vi "Control Experiment.vi"(8 "Error In":errorcluster, 9 "KH":T5={"KH #"=[0, 1, 2, 3, 4, 5, 6, 7, 8, 9, 10, 11, 12, 13, 14, 15], "KH Configuration"=[enum."SE+ (-gnd)", enum."SE+ (-gnd)", enum."Differential", enum."Differential", enum."SE+ (-gnd)", enum."Differential", enum."Differential", enum."SE+ (-gnd)", enum."Differential", enum."Differential", enum."SE+ (-gnd)", enum."SE+ (-gnd)", enum."Differential", enum."Ground", enum."Ground", enum."Ground"], "KH Gain"=[enum."1000x", enum."1000x", enum."1000x", enum."1000x", enum."1000x", enum."1000x", enum."1000x", enum."1000x", enum."1000x", enum."1000x", enum."1000x", enum."1000x", enum."1000x", enum."100x", enum."100x", enum."100x"], "KH Shunt Resistor"=[enum."Open", enum."Open", enum."5k Ohms", enum."5k Ohms", enum."Open", enum."5k Ohms", enum."5k Ohms", enum."Open", enum."5k Ohms", enum."5k Ohms", enum."Open", enum."Open", enum."50k Ohms", enum."Open", enum."Open", enum."Open"]} {"KH #" items=["A 1", "A 2", "A 3", "A 4", "A 5", "A 6", "A 7", "A 8", "B 1", "B 2", "B 3", "B 4", "B 5", "B 6", "B 7", "B 8"]}, 10 "Lockin":T7={"AI"=[1, 2, 3, 4, 5, 6, 7, 8, 9, 10, 11, 12, 13, 14, 15, 16], "Electrode"=["4", "5", "6", "7", "9", "11", "12", "13", "16", "17", "20", "21", "1", "", "", ""], "Label"=[8, 8, 9, 9, 8, 9, 9, 8, 2, 1, 3, 4, 6, 0, 0, 0], "Electrode Config"=[enum."Voltage (SE)", enum."Voltage (SE)", enum."Current", enum."Current", enum."Voltage (SE)", enum."Current", enum."Current", enum."Voltage (SE)", enum."Current", enum."Current", enum."Voltage (SE)", enum."Voltage (SE)", enum."Gate", enum."Ground", enum."Ground", enum."Ground"]} {"Label" items=["", "I+", "I-", "V1+", "V1-", "dV1", "Vsg", "Vbg", "V2", "I2", "I3", "V3"]}) -> (0 "Error Out":errorcluster)   [LabVIEW 2016, in "Control Experiment SM.lvclass"]
doc: "Use this VI to help configure your experiment.\n1. Choose Pickering or Not Pickering\n2. Configure the Electrode control to show which electrode is connected to which lockin\n3. Choose a Label for each electrode to configure Krohn Hite amplifier automatically\n4. Easily set all Krohn Hite channels to be \"all ground\" or \"all differential\" mode\n5. Fill out information about you and your device in the lower left corner\n6. When you are finished, or when you want to update the amplifiers, click the \"CREATE OUTPUT\" button located in upper right. Clicking this button will set the amplifiers, Pickering switch (if you have one), and write information to a functional global variable that you can easily read from elsewhere in your program"
uses:
  Control Experiment SM.lvclass
  <vilib>/addons/_JKI.lib/Serialization/JSON/JKI JSON Serialization.lvlib
  Typedefs/KH Mode-enum.ctl
  <userlib>/LevyLab/Krohn Hite 7008/typedefs/Gain-Enum.ctl
  <userlib>/LevyLab/Krohn Hite 7008/Instrument.KH7008.lvclass
  <userlib>/LevyLab/Krohn Hite 7008/typedefs/Shunt-Enum.ctl
  <userlib>/LevyLab/Krohn Hite 7008/typedefs/Input Configuration-Enum.ctl
  <vilib>/addons/_JKI.lib/REST Client/classes/REST Client/HTTP Header.ctl
  <vilib>/addons/_JKI.lib/REST Client/classes/REST Client/REST Client.lvclass
  <vilib>/JKI/JKI SMO/SMO/SMO.lvclass
  Typedefs/Control Experiment JSON--cluster.ctl
  <vilib>/Utility/sysdir.llb/System Directory Type.ctl
  <userlib>/LevyLab/Levylab Instruments/SMOs/Configuration/Configuration.lvclass
  Typedefs/Instrument--enum.ctl
  Typedefs/UI Controls --cluster.ctl
  <userlib>/_OpenG.lib/array/array.llb/Remove Duplicates from 1D Array (Variant)__ogtk.vi
  <userlib>/LevyLab/Krohn Hite 7008/typedefs/Channel-Enum.ctl
  <userlib>/LevyLab/Krohn Hite 7008/typedefs/Filter-Enum.ctl
  <userlib>/LevyLab/Krohn Hite 7008/typedefs/Coupling-Enum.ctl
  <userlib>/LevyLab/Krohn Hite 7008/typedefs/SetAll-Cluster.ctl
  <userlib>/LevyLab/Krohn Hite 7008/typedefs/SetAll-Array.ctl
  <userlib>/LevyLab/Levylab Instruments/SMOs/Logger.PGSQL/Logger.PGSQL.lvclass
  <userlib>/LevyLab/Lockin-Multichannel/Instrument.Lockin/Instrument.Lockin.lvclass
  <userlib>/LevyLab/Levylab Instruments/Instrument Types/CBridge/Instrument.CBridge.lvclass
  <userlib>/LevyLab/Levylab Instruments/Instrument Types/Strain/Instrument.Strain.lvclass
  <userlib>/_MGI/File/MGI Create Directory Chain Behavior Enum.ctl
  C:/Program Files (x86)/National Instruments/LabVIEW 2016/user.lib/LevyLab/Levylab Instruments/SMOs/Logger/Logger.lvclass
  C:/Program Files (x86)/National Instruments/LabVIEW 2016/vi.lib/JKI/JKI SMO/SMO/SMO.lvclass
panel:
  in  "I'm Finished Taking Data!":bool
  out "Values have changed":bool=TRUE
  in  "Create Output":bool
  in  "OK":bool
  out "Control Experiment":refnum<class "Control Experiment SM.lvclass">
  in  "C.E.":refnum<class "Control Experiment SM.lvclass">
  in  "Tab Control":T1(tab)=enum."Sandbox"
  in  "DC Coupled":bool=TRUE
  in  "Bandwidth Filter":bool=TRUE
  in  "#AO":u32=8
  in  "Gain":dbl[](array[numeric])=[1.0, 1.0, 1.0, 1.0, 1.0, 1.0, 1.0, 1.0, 1.0, 1.0, 1.0, 1.0, 1.0, 1.0, 1.0, 1.0]
  in  "#AI":u32=16
  in  "KH All Buttons":T8(radio)
  in  "Defualt Shunt Resistor":T4=enum."5k Ohms"
  in  "Description":string="    devices:\n    \n    1. 80x80um rectangle\n    2. hash: 200 horizontal and vertical lines 400nm apart\n    3. hash structures: 400, 200nm apart horizontal and vertical lines"
  in  "Sample (SAXXXX)":string="SA40178"
  in  "Device (YYYYMMDD)":string="20210125"
  in  "Instrument":T9=enum."MNK"
  in  "Username":string="Aditi"
  in  "non KH":T10 {"Labels 2" items=["", "I+", "I-", "V1+", "V1-", "dV1", "Vsg", "Vbg", "V2", "I2", "I3", "V3"]}
  in  "Strain Cell Address":refnum<visa-resource-name>
  in  "Capacitance Bridge Address":refnum<visa-resource-name>
  in  "C Bridge?":bool
  in  "Strain Cell?":bool
  in  "Krohn Hite?":bool=TRUE
  in  "KH Addresses":refnum<visa-resource-name>[](array[refnum])=["COM20", "COM14"] caption="KH Address[A,B,C,...]"
  in  "Lockin Address":string
  in  "Ring":u16(ring)=2 items=["----Sweep Control----", "Sweep Control.vi", "Continuous B Sweep.vi", "----Transport----", "IV.vi", "IV_Sweep.vi", "Lockin_time.vi", "Lockin_Vsg.vi", "Lockin_sweep.vi", "Lockin_AIWFM_time.vi", "THz_TimeDelay.vi", "Sweep_AIWFM_time.vi"]
  in  "Open VI":bool
  in  "Open Lockin":bool
  in  "Write Pickering Config":bool
  in  "Read Pickering Config":bool
  out "Refresh Token Out":string="0/0ccae0b202a2d5ce21e5be9cd72246b8"
  in  "Default Path":path=path "D:/Data" caption="Default Path (Do not add your instrument name here)(Typ. G:\\My Drive\\ansom\\Data)"
  out "Comments":string="Device: \r  Device Name: SA40178.20210125\r  Computer: KHOLEK\r  User: Aditi\r  Instrument: MNK\r  Description: |\r        devices:\r        \r        1. 80x80um rectangle\r        2. hash: 200 horizontal and vertical lines 400nm apart\r        3. hash structures: 400, 200nm apart horizontal and vertical lines\r\rExperiment: \r  Time: 2021-02-22T11:02:02\r  Description: |\r\rSweep: \r- Loop1: [OFF, 0.000000]\r- Loop2: [OFF, 0.000000]\r- Loop3: [OFF, 0.000000]\r- Loop4: [OFF, 0.000000]\r\rWiring: \r- Electrode 4: Lockin 1, V2, KH1 Channel 1, SE+ (-gnd), 1000x, Open\r- Electrode 5: Lockin 2, V2, KH1 Channel 2, SE+ (-gnd), 1000x, Open\r- Electrode 6: Lockin 3, I2, KH1 Channel 3, Differential, 1000x, 5k Ohms\r- Electrode 7: Lockin 4, I2, KH1 Channel 4, Differential, 1000x, 5k Ohms\r- Electrode 9: Lockin 5, V2, KH1 Channel 5, SE+ (-gnd), 1000x, Open\r- Electrode 11: Lockin 6, I2, KH1 Channel 6, Differential, 1000x, 5k Ohms\r- Electrode 12: Lockin 7, I2, KH1 Channel 7, Differential, 1000x, 5k Ohms\r- Electrode 13: Lockin 8, V2, KH1 Channel 8, SE+ (-gnd), 1000x, Open\r- Electrode 16: Lockin 9, I-, KH2 Channel 1, Differential, 1000x, 5k Ohms\r- Electrode 17: Lockin 10, I+, KH2 Channel 2, Differential, 1000x, 5k Ohms\r- Electrode 20: Lockin 11, V1+, KH2 Channel 3, SE+ (-gnd), 1000x, Open\r- Electrode 21: Lockin 12, V1-, KH2 Channel 4, SE+ (-gnd), 1000x, Open\r- Electrode 1: Lockin 13, Vsg, KH2 Channel 5, Differential, 1000x, 50k Ohms\r\rLockin: \r  AO: \r  - AO 1: amp = 0.000 mV, DC = 0.000 mV, f = 1.00 Hz, phi = 0.00°, Triangle\r  - AO 2: amp = 0.000 mV, DC = 0.000 mV, f = 1.00 Hz, phi = 0.00°, Triangle\r  - AO 3: amp = 0.000 mV, DC = 0.000 mV, f = 1.00 Hz, phi = 0.00°, Triangle\r  - AO 4: amp = 0.000 mV, DC = 0.000 mV, f = 1.00 Hz, phi = 0.00°, Triangle\r  - AO 5: amp = 0.000 mV, DC = 0.000 mV, f = 1.00 Hz, phi = 0.00°, Triangle\r  - AO 6: amp = 10.000 mV, DC = 0.000 mV, f = 1.00 Hz, phi = 0.00°, Triangle\r  - AO 7: amp = 0.000 mV, DC = 0.000 mV, f = 1.00 Hz, phi = 0.00°, Triangle\r  - AO 8: amp = 0.000 mV, DC = 0.000 mV, f = 1.00 Hz, phi = 0.00°, Triangle\r  - AO 9: amp = 0.000 mV, DC = 0.000 mV, f = 1.00 Hz, phi = 0.00°, Triangle\r  - AO 10: amp = 10.000 mV, DC = 0.000 mV, f = 1.00 Hz, phi = 0.00°, Triangle\r  - AO 11: amp = 0.000 mV, DC = 0.000 mV, f = 1.00 Hz, phi = 0.00°, Triangle\r  - AO 12: amp = 0.000 mV, DC = 0.000 mV, f = 1.00 Hz, phi = 0.00°, Triangle\r  - AO 13: amp = 0.000 mV, DC = 0.000 mV, f = 1.00 Hz, phi = 0.00°, Sine\r  - AO 14: amp = 0.000 mV, DC = 0.000 mV, f = 1.00 Hz, phi = 0.00°, Sine\r  - AO 15: amp = 0.000 mV, DC = 0.000 mV, f = 1.00 Hz, phi = 0.00°, Sine\r  - AO 16: amp = 0.000 mV, DC = 0.000 mV, f = 1.00 Hz, phi = 0.00°, Sine\r  - AO 17: amp = 0.000 mV, DC = -0.000 mV, f = 1.00 Hz, phi = 0.00°, Sine\r  - AO 18: amp = 0.000 mV, DC = 0.000 mV, f = 1.00 Hz, phi = 0.00°, Sine\r  - AO 19: amp = 0.000 mV, DC = 0.000 mV, f = 1.00 Hz, phi = 0.00°, Sine\r  - AO 20: amp = 0.000 mV, DC = 0.000 mV, f = 1.00 Hz, phi = 0.00°, Sine\r  - AO 21: amp = 0.000 mV, DC = 0.000 mV, f = 1.00 Hz, phi = 0.00°, Sine\r  - AO 22: amp = 0.000 mV, DC = 0.000 mV, f = 1.00 Hz, phi = 0.00°, Sine\r  - AO 23: amp = 0.000 mV, DC = 0.000 mV, f = 1.00 Hz, phi = 0.00°, Sine\r  - AO 24: amp = 0.000 mV, DC = 0.000 mV, f = 1.00 Hz, phi = 0.00°, Sine\r  REF: \r  - Lockin 1: f = 1.00 Hz, phi = 0.00°, TC = 0.10 s, order = 2 \r  Sampling: \r  - Fs: 10000.000000\r  - N: 1000\r"
  out "Device Folder":path=path "D:/Data/MNK/SA40178.20210125" caption="(\\base path\\project\\device\\ )"
  out "JSON String":string="{\r\n    \"Device\":{\r\n        \"Device\":\"SA40178.20210125\",\r\n        \"User\":\"Aditi\",\r\n        \"Time\":\"2021-02-22T11:02:02\",\r\n        \"Computer Name\":\"KHOLEK\"\r\n    },\r\n    \"Wiring\":{\r\n        \"Lockin Ch\":[\r\n            1,\r\n            2,\r\n            3,\r\n            4,\r\n            5,\r\n            6,\r\n            7,\r\n            8,\r\n            9,\r\n            10,\r\n            11,\r\n            12,\r\n            13,\r\n            14,\r\n            15,\r\n            16\r\n        ],\r\n        \"KH Electrodes\":[\r\n            \"4\",\r\n            \"5\",\r\n            \"6\",\r\n            \"7\",\r\n            \"9\",\r\n            \"11\",\r\n            \"12\",\r\n            \"13\",\r\n            \"16\",\r\n            \"17\",\r\n            \"20\",\r\n            \"21\",\r\n            \"1\",\r\n            \"\",\r\n            \"\",\r\n            \"\"\r\n        ],\r\n        \"KH Labels\":[\r\n            \"V2\",\r\n            \"V2\",\r\n            \"I2\",\r\n            \"I2\",\r\n            \"V2\",\r\n            \"I2\",\r\n            \"I2\",\r\n            \"V2\",\r\n            \"I-\",\r\n            \"I+\",\r\n            \"V1+\",\r\n            \"V1-\",\r\n            \"Vsg\",\r\n            \"\",\r\n            \"\",\r\n            \"\"\r\n        ],\r\n        \"Other Electrodes\":[\r\n            \"4\",\r\n            \"5\",\r\n            \"6\",\r\n            \"7\",\r\n            \"9\",\r\n            \"11\",\r\n            \"12\",\r\n            \"13\",\r\n            \"16\",\r\n            \"17\",\r\n            \"20\",\r\n            \"21\",\r\n            \"1\",\r\n            \"\",\r\n            \"\",\r\n            \"\"\r\n        ],\r\n        \"Other Labels\":[\r\n            \"V2\",\r\n            \"V2\",\r\n            \"I2\",\r\n            \"I2\",\r\n            \"V2\",\r\n            \"I2\",\r\n            \"I2\",\r\n            \"V2\",\r\n            \"I-\",\r\n            \"I+\",\r\n            \"V1+\",\r\n            \"V1-\",\r\n            \"Vsg\",\r\n            \"\",\r\n            \"\",\r\n            \"\"\r\n        ]\r\n    }\r\n}"
  in  "Labels Strings":string[](array[string])=["", "I+", "I-", "V1+", "V1-", "dV1", "Vsg", "Vbg", "V2", "I2", "I3", "V3"]
  out "YAML example":string="description: This is a dummy dataset which mimics smFRET data.\n\nsetup:\n    ## Mandatory fields\n    num_pixels: 2                # using 2 detectors\n    num_spots: 1                 # a single confocal excitation\n    num_spectral_ch: 2           # donor and acceptor detection\n    num_polarization_ch: 1       # no polarization selection\n    num_split_ch: 1              # no beam splitter\n    modulated_excitation: False  # CW excitation, no modulation\n    lifetime: False              # no TCSPC in detection\n\n    ## Optional fields\n    excitation_wavelengths:      # List of excitation wavelenghts\n       - !!float 532e-9\n    excitation_cw:               # List of booleans, True if wavelength is CW\n       - True\n    detection_wavelengths:       # Nominal center wavelength for each for detection ch\n       - !!float 580e-9\n       - !!float 640e-9\n\nsample:\n  sample_name: describe the sample here\n  buffer_name: describe the buffer here\n  dye_names: 'Cy3B, ATTO647N'   # Comma separates names of fluorophores\n\nidentity:\n    author: Author Name\n    author_affiliation: Name of Research Institution\n\nprovenance:\n    filename: 'photon_data.hdf5'\n    software: Acquisition Software Name\n\nphoton_data:\n    timestamps_specs:\n        timestamps_unit: !!float 10e-9  # 10 ns\n    measurement_specs:\n        measurement_type: smFRET\n        detectors_specs:\n            spectral_ch1: [0]  # list of donor's detector IDs\n            spectral_ch2: [1]  # list of acceptor's detector IDs"
  in  "String":string
  # "SANDBOX:"
  # "Sample"
  # "Krohn Hite"
  # "Lockin"
  # "Lockin"
  # "Krohn Hite"
  # "Other"
  # "Device and Project Description"
  # "Hardware Configuration"
  # "Experiment VIs"
  # "Lockin (Local)"
  # "Path Configuration"
  # "Use this VI to help configure your experiment.\n1. Choose Pickering or Not Pickering\n2. Configure the Electrode control to show which electrode is connected to which lockin\n3. Choose a Label for each electrode to configure Krohn Hite amplifier automatically\n4. Easily set all Krohn Hite channels to be \"all ground\" or \"all differential\" mode\n5. Fill out information about you and your device in the lower left corner\n6. When you are finished, or when you want to update the amplifiers, click the \"CREATE OUTPUT\" button located in upper right.\nClicking this button will set the amplifiers, Pickering switch (if you have one), and write information to a functional global variable that you can easily read from elsewhere in your program"
  # "If you want to have new labels for the \"Labels\" field you can type them here"
  # "The magic words are:\nI\nVsg\nVbg\ndV\nV"
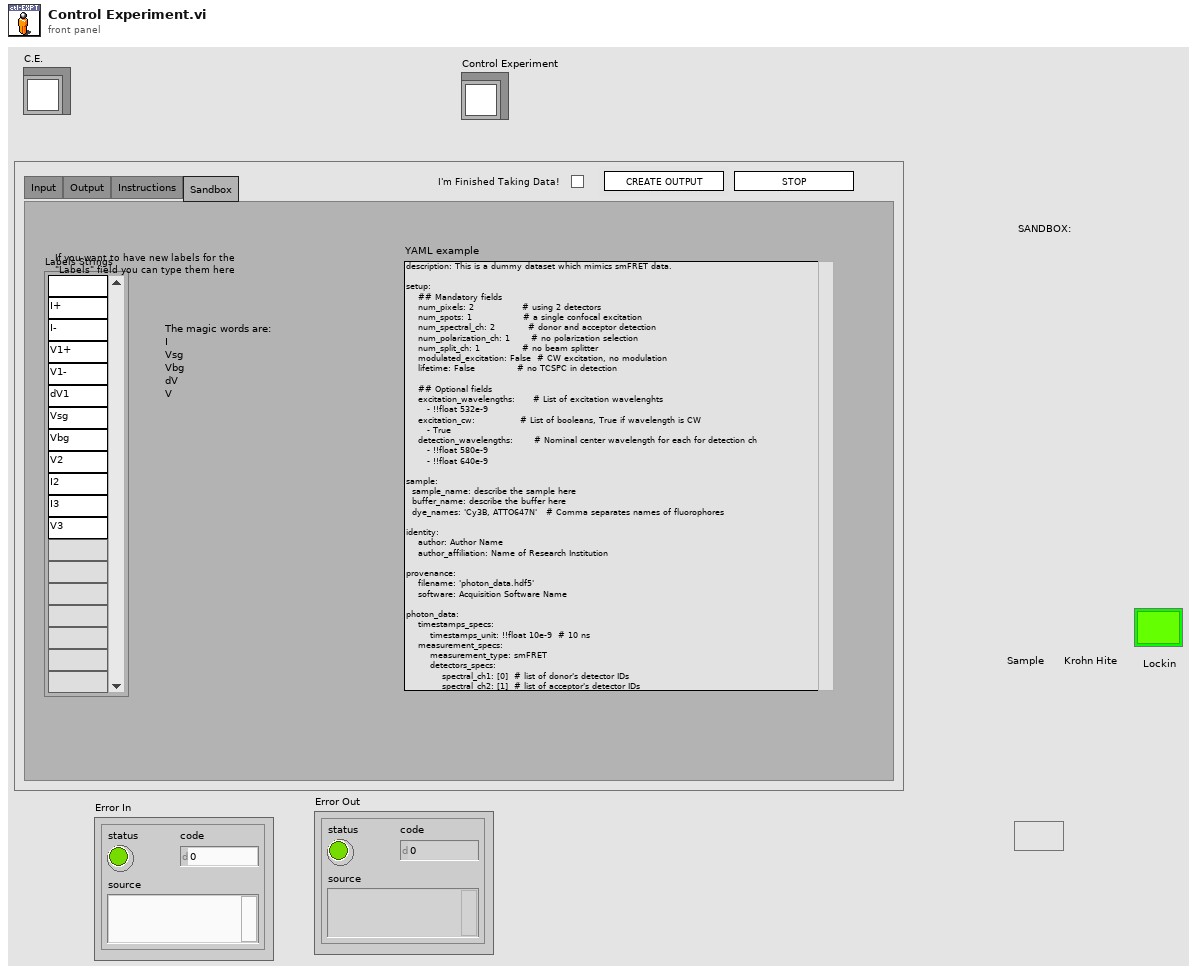
[diagram p1: front panel]
types:
  T1 = enum32{"Input", "Pickering", "Output", "Instructions", "Sandbox"}
  T2 = typedef "Instrument.KH7008.lvclass/Input Configuration-Enum.ctl" = enum16{"Ground", "SE+ (-gnd)", "SE- (+gnd)", "Differential"}
  T3 = typedef "Instrument.KH7008.lvclass/Gain-Enum.ctl" = enum16{"1x", "10x", "100x", "1000x"}
  T4 = typedef "Instrument.KH7008.lvclass/Shunt-Enum.ctl" = enum16{"Open", "50 Ohms", "500 Ohms", "5k Ohms", "50k Ohms", "10M Ohm"}
  T5 = cluster{"KH #":u16[], "KH Configuration":T2[], "KH Gain":T3[], "KH Shunt Resistor":T4[]}
  T6 = typedef "Control Experiment SM.lvclass/KH Mode-enum.ctl" = enum16{"Ground", "Current", "Voltage (SE)", "Voltage (Diff)", "Gate"}
  T7 = cluster{"AI":u32[], "Electrode":string[], "Label":u16[], "Electrode Config":T6[]}
  T8 = enum32{"No Selection", "All Ground", "All Differential"}
  T9 = typedef "Control Experiment SM.lvclass/Instrument--enum.ctl" = enum16{"----- AFM/EBL -----", "AGILENT", "CYPHER", "Gemini2", "JEOL", "MFP3D", "----- Cryostat -----", "CF900", "DR200", "MNK", "PPMS 1", "PPMS 2", "PPMS 3", "----- Optics -----", "THz 1", "THz 2"}
  T10 = cluster{"Scroll Bar":string[], "Electrodes 2":string[], "Labels 2":u16[], "unused":string[]}
  T11 = enum16{"A 1", "A 2", "A 3", "A 4", "A 5", "A 6", "A 7", "A 8", "B 1", "B 2", "B 3", "B 4", "B 5", "B 6", "B 7", "B 8", "none"}
  T12 = enum32{"invalid app kind", "Development System", "Run Time System", "Student Edition", "Embedded LabVIEW", "Evaluation", "Custom"}
  T13 = enum32{"Bad", "Idle", "Run top level", "Running"}
  T14 = enum32{"Invalid", "Standard", "Closed", "Hidden", "Minimized", "Maximized"}
  T15 = typedef "MGI Create Directory Chain Behavior Enum.ctl" = enum16{"Auto Detect", "Path Contains a File", "Path Does Not Contain a File"}
  T16 = typedef "Instrument.KH7008.lvclass/SetAll-Cluster.ctl" = cluster{"Channel":T17, "Gain":T3, "Bandwidth Filter":T18, "Shunt Resistor":T4, "Coupling":T19, "Input Config":T2}
  T17 = typedef "Instrument.KH7008.lvclass/Channel-Enum.ctl" = enum16{"Channel 1", "Channel 2", "Channel 3", "Channel 4", "Channel 5", "Channel 6", "Channel 7", "Channel 8"}
  T18 = typedef "Instrument.KH7008.lvclass/Filter-Enum.ctl" = enum16{"OFF", "ON"}
  T19 = typedef "Instrument.KH7008.lvclass/Coupling-Enum.ctl" = enum16{"AC", "DC"}
  T20 = enum16{"GSR", "Research Projects", "Undergrads", "Researchers", "Hardware", "Software", "LevyLab", "Samples", "Manuscripts", "AoT", "WorkStudy"}
  T21 = enum16{"A 1", "A 2", "A 3", "A 4", "A 5", "A 6", "A 7", "A 8", "B 1", "B 2", "B 3", "B 4", "B 5", "B 6", "B 7", "B 8", "none"}[]
  T22 = typedef "Control Experiment SM.lvclass/Experiment Description--cluster.ctl" = cluster{"User":string, "Device":string, "Device Path":path, "Device Description":string, "Experiment Path":path, "Experiment Description":string, "Instrument":T9, "Device Description (JSON)":string, "Experiment Description (JSON)":string, "Comments":string, "Sweep":cluster{"key":string, "value":variant}[]}
  T23 = typedef "Control Experiment SM.lvclass/Wiring Description--cluster.ctl" = cluster{"AI":cluster{"Channel":u32, "Gain":dbl}, "Device":cluster{"Electrode":string, "Label":string, "Type":string}, "KH":cluster{"Channel":string, "Configuration":string, "Gain":u32, "Shunt Resistor":u32}, "AO":cluster{"Channel":u32, "Gain":dbl}}[]
  T24 = typedef "Instrument.KH7008.lvclass/SetAll-Array.ctl" = T16[]
  T25 = typedef "Control Experiment SM.lvclass/UI Controls --cluster.ctl" = cluster{"Sample":string, "Device":string, "Username":string, "Description":string, "Default Path":path, "AWS Path":path, "Instrument":T9, "Lockin?":bool, "Lockin Address":string, "Krohn Hite?":bool, "KH Addresses":refnum<visa-resource-name>[], "KH All Buttons":enum32{"No Selection", "All Ground", "All Differential"}, "Strain Cell?":bool, "Strain Cell Address":refnum<visa-resource-name>, "C Bridge?":bool, "Capacitance Bridge Address":refnum<visa-resource-name>, "Lockin":cluster{"AI":u32[], "Electrode":string[], "Label":u16[], "Electrode Config":T6[]}, "KH":cluster{"KH #":enum16{"A 1", "A 2", "A 3", "A 4", "A 5", "A 6", "A 7", "A 8", "B 1", "B 2", "B 3", "B 4", "B 5", "B 6", "B 7", "B 8", "none"}[], "KH Configuration":T2[], "KH Gain":T3[], "KH Shunt Resistor":T4[], "Filter":bool, "DC Coupled":bool}, "non KH":cluster{"Scroll Bar":string[], "Electrodes 2":string[], "Labels 2":u16[], "unused":string[]}, "#AI":u32}
  T26 = typedef "REST Client.lvlib/REST Client.lvclass/HTTP Header.ctl" = cluster{"header":string, "value":string}
  T27 = cluster{"Core":cluster{"Current VI Reference":refnum<vi>, "Close Panel on Exit?":bool}, "C.E.":refnum<class "Control Experiment SM.lvclass">, "Experiment":T22, "Wiring":T23, "Channel Settings":cluster{"Channel Setting":T24}[], "KH All Buttons":enum32{"No Selection", "All Ground", "All Differential"}, "Lockin":cluster{"AI":u32[], "Electrode":string[], "Label":u16[], "Electrode Config":T6[]}, "KH":cluster{"KH #":u16[], "KH Configuration":T2[], "KH Gain":T3[], "KH Shunt Resistor":T4[]}, "non KH":cluster{"Scroll Bar":string[], "Electrodes 2":string[], "Labels 2":u16[], "unused":string[]}, "UI":T25, "Asana":cluster{"Authentication Info":cluster{"Client ID":string, "Client Secret":string, "Redirect URI":string, "Token Endpoint":string, "Scope":string}, "Authentication Header":T26[], "Refresh Token":string, "Time Stamp":timestamp}, "Logger":refnum<class "Logger.PGSQL.lvclass">, "Config":refnum<class "Configuration.lvclass">, "VI paths":path[], "top level?":bool}
  T28 = cluster{"Authentication Info":cluster{"Client ID":string, "Client Secret":string, "Redirect URI":string, "Token Endpoint":string, "Scope":string}, "Authentication Header":T26[], "Refresh Token":string, "Time Stamp":timestamp}
  T29 = cluster{"Current VI Reference":refnum<vi>, "Close Panel on Exit?":bool}
  T30 = typedef "System Directory Type.ctl" = i32
  T31 = typedef "Control Experiment SM.lvclass/Control Experiment JSON--cluster.ctl" = cluster{"Device":cluster{"Device":string, "User":string, "Time":string, "Computer Name":string}, "Wiring":cluster{"Lockin Ch":u32[], "KH Electrodes":string[], "KH Labels":string[], "Other Electrodes":string[], "Other Labels":string[]}}
  T32 = cluster{"Client ID":string, "Client Secret":string, "Redirect URI":string, "Token Endpoint":string, "Scope":string}
  T33 = cluster{"gid":string, "name":string, "resource_type":string}[]
  T34 = cluster{"id":i64, "gid":string, "resource_type":string, "name":string}[]
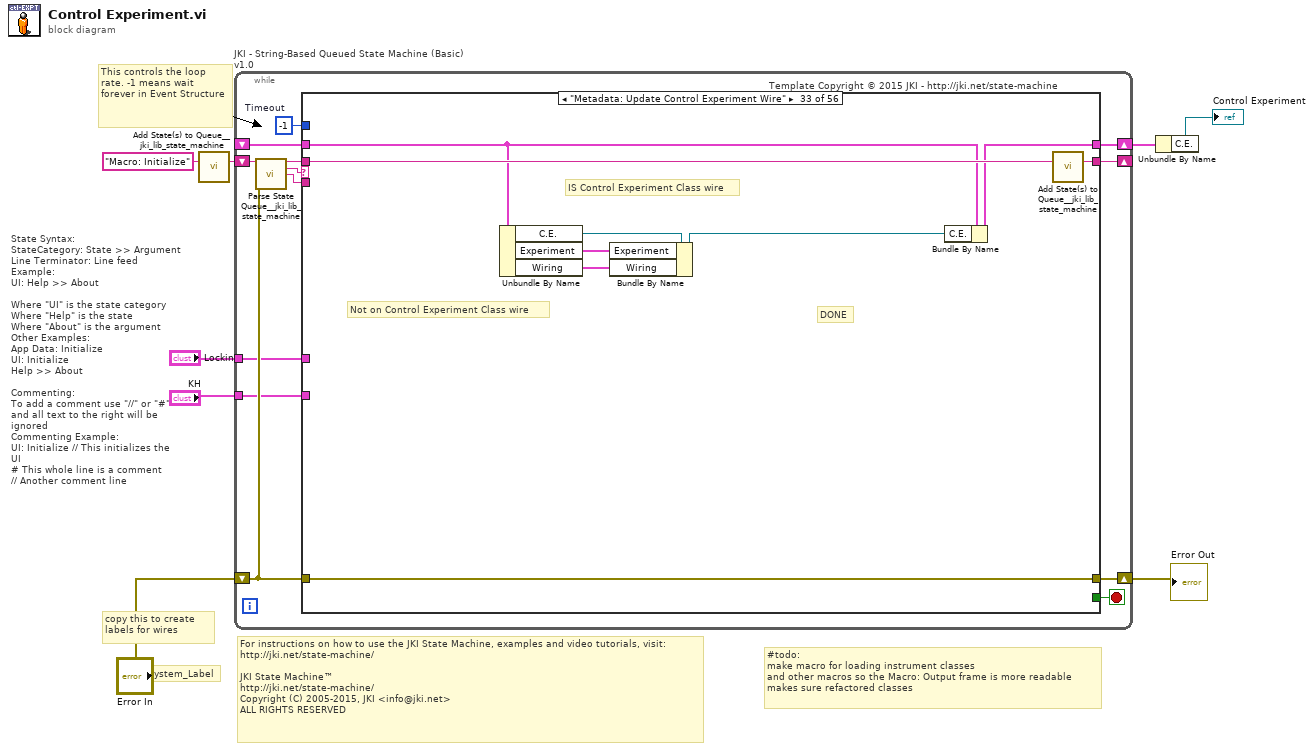
[diagram p0: block diagram]
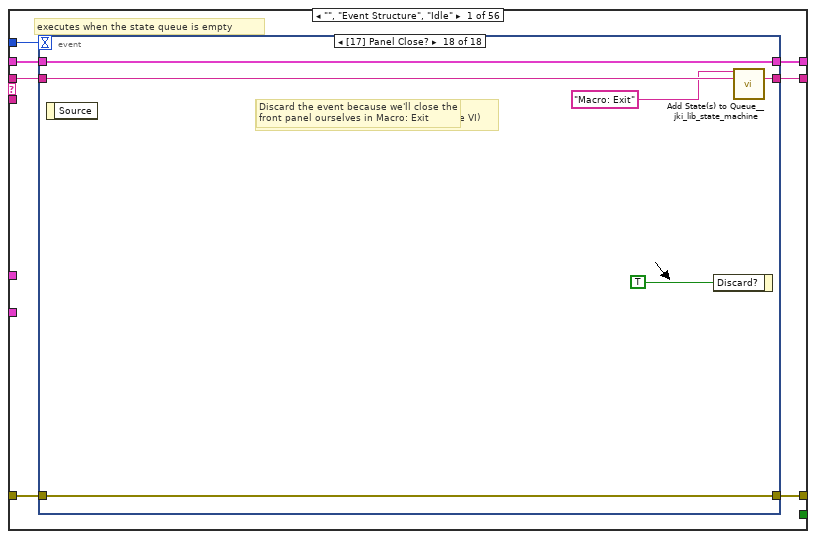
[diagram p2: hidden frame]
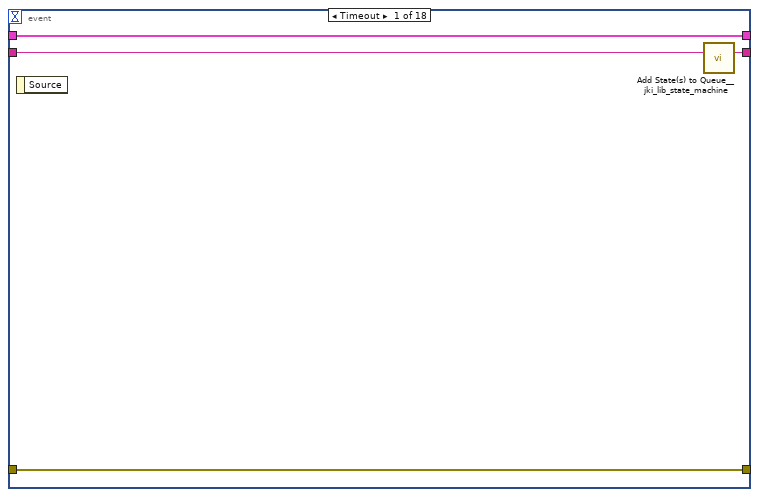
[diagram p3: hidden frame]
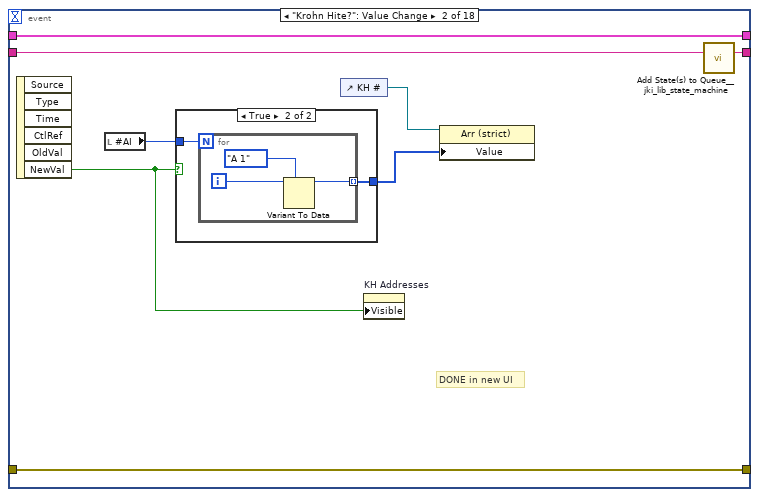
[diagram p4: hidden frame]
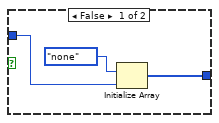
[diagram p5: hidden frame]
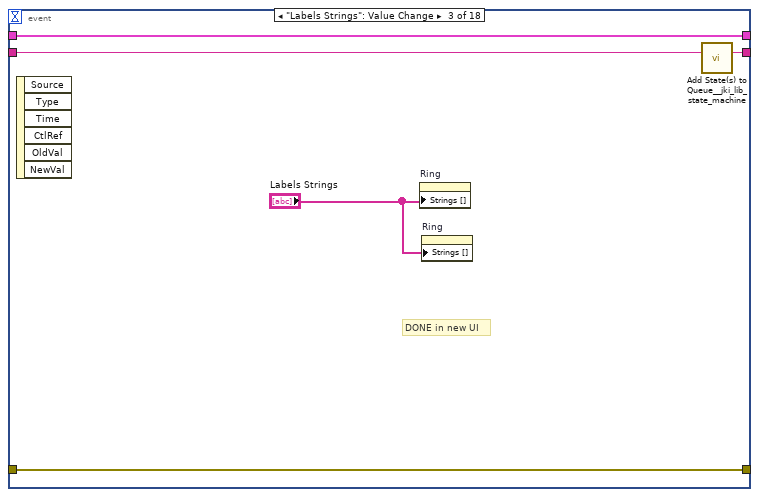
[diagram p6: hidden frame]
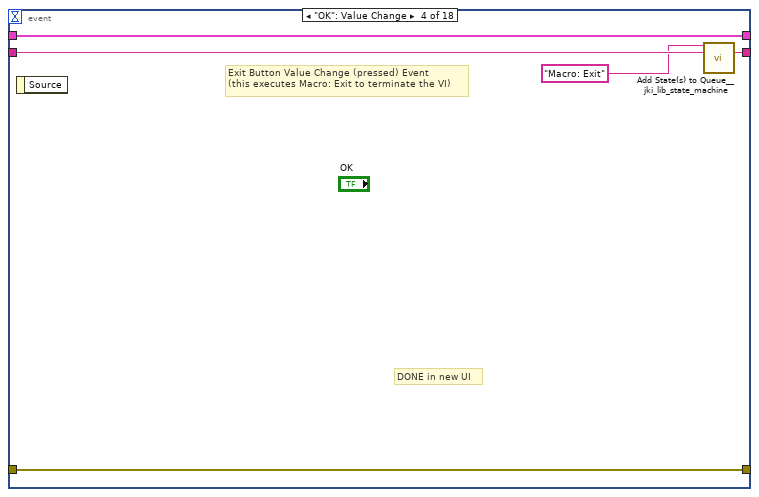
[diagram p7: hidden frame]
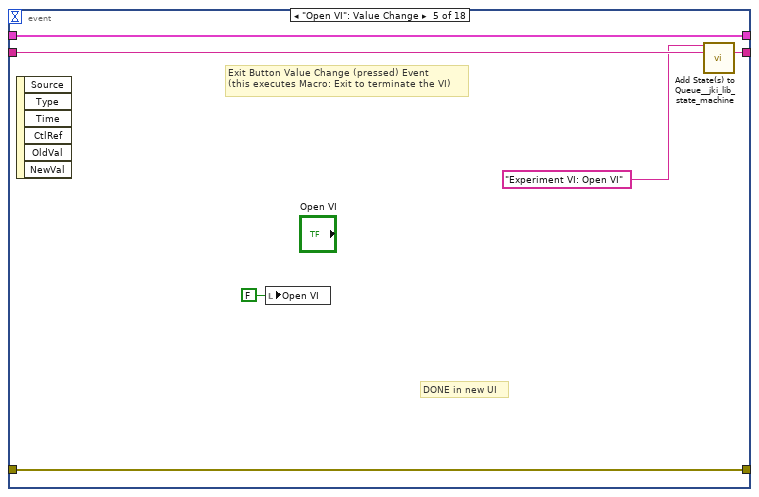
[diagram p8: hidden frame]
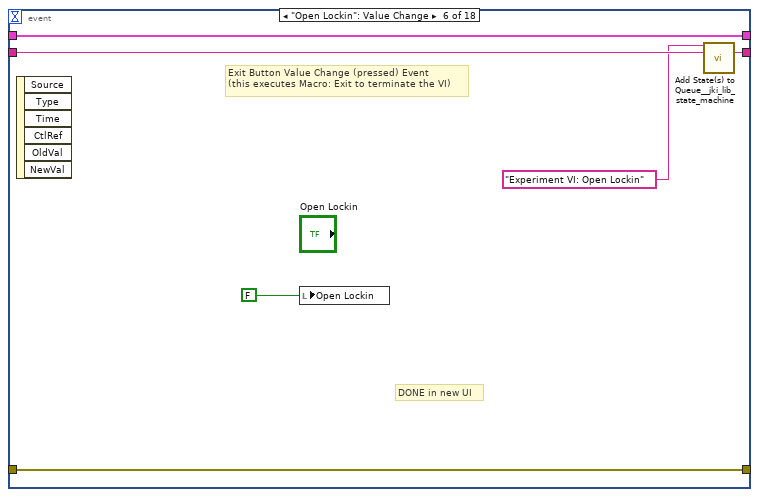
[diagram p9: hidden frame]
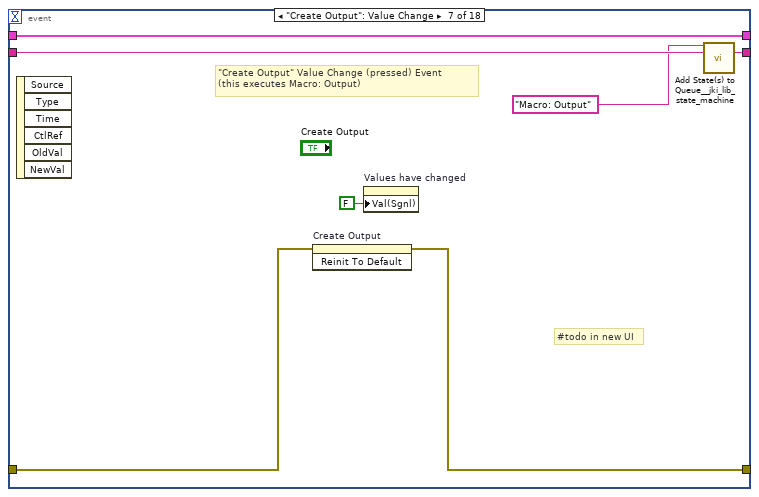
[diagram p10: hidden frame]
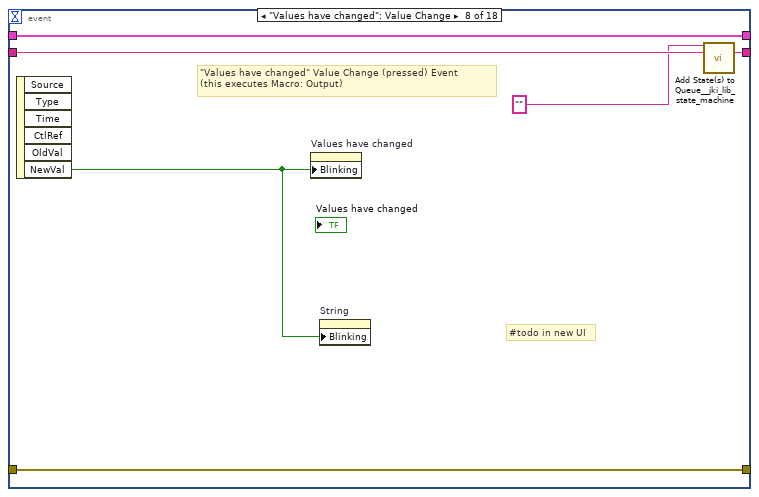
[diagram p11: hidden frame]
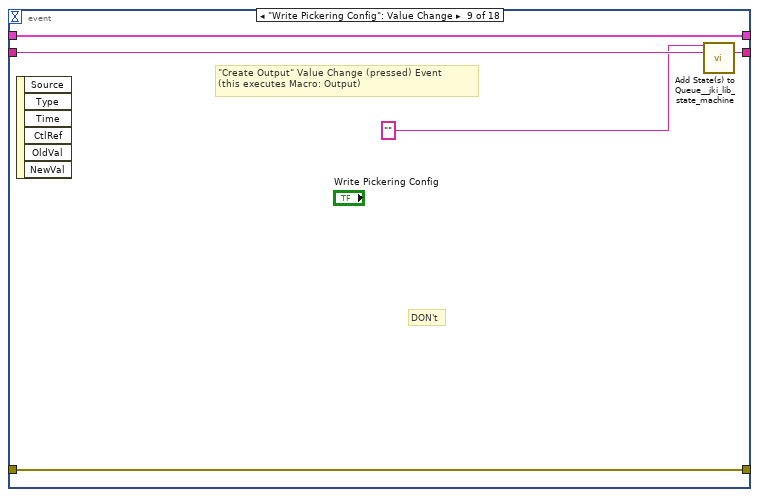
[diagram p12: hidden frame]
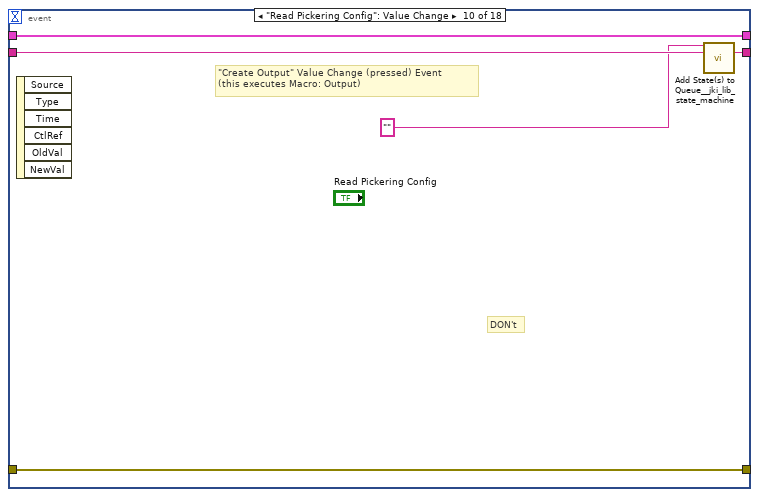
[diagram p13: hidden frame]
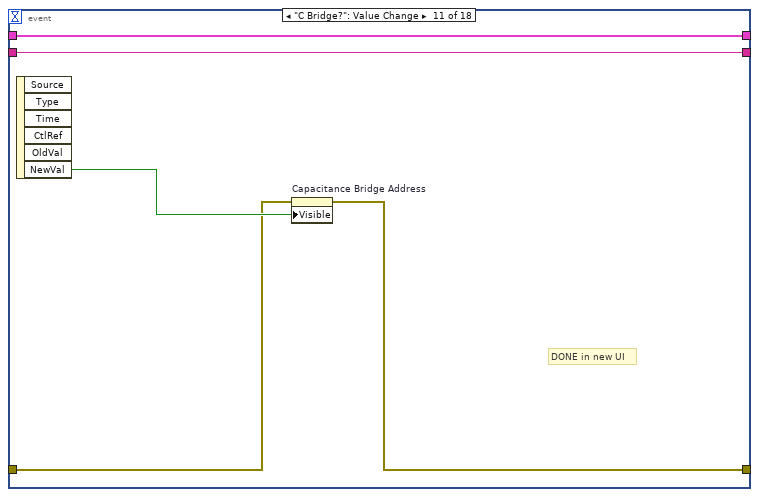
[diagram p14: hidden frame]
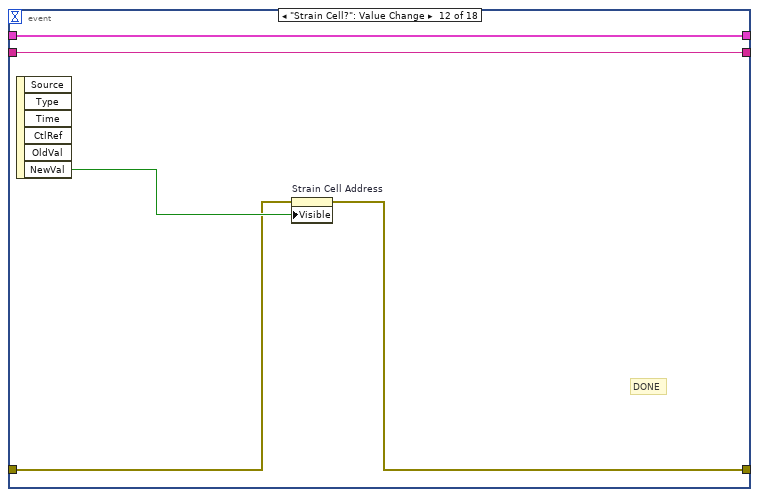
[diagram p15: hidden frame]
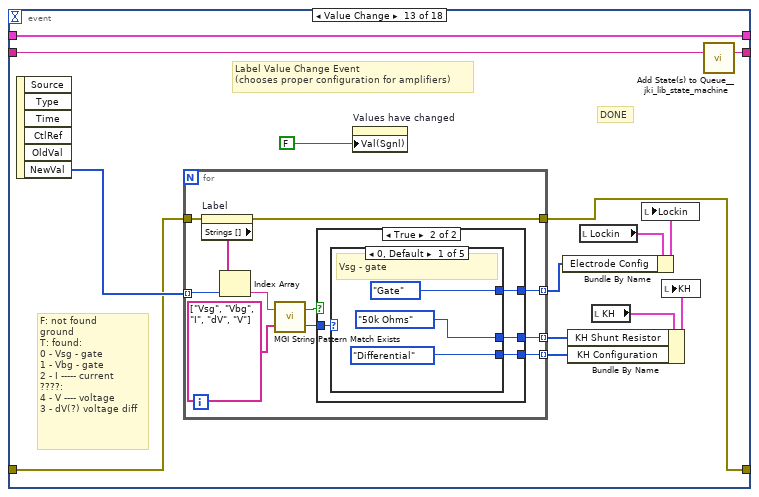
[diagram p16: hidden frame]
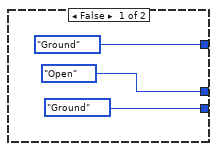
[diagram p17: hidden frame]
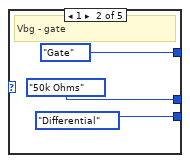
[diagram p18: hidden frame]
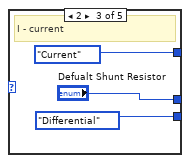
[diagram p19: hidden frame]
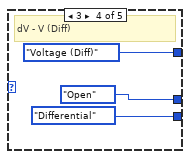
[diagram p20: hidden frame]
diagram:
  # "#todo:\nmake macro for loading instrument classes\nand other macros so the Macro: Output frame is more readable\nmakes sure refactored classes"
  # "For instructions on how to use the JKI State Machine, examples and video tutorials, visit:\nhttp://jki.net/state-machine/\n\nJKI State Machine™\nhttp://jki.net/state-machine/\nCopyright (C) 2005-2015, JKI <info@jki.net>\nALL RIGHTS RESERVED"
  # "State Syntax:\nStateCategory: State >> Argument\nLine Terminator: Line feed\nExample:\nUI: Help >> About\n\nWhere \"UI\" is the state category\nWhere \"Help\" is the state\nWhere \"About\" is the argument\nOther Examples:\nApp Data: Initialize\nUI: Initialize\nHelp >> About\n\nCommenting:\nTo add a comment use \"//\" or \"#\" and all text to the right will be ignored\nCommenting Example:\nUI: Initialize // This initializes the UI\n# This whole line is a comment\n// Another comment line"
  # "copy this to create labels for wires"
  # "This controls the loop rate. -1 means wait forever in Event Structure"
  # "System_Label"
  n1 = call <vilib>:"Add State(s) to Queue__jki_lib_state_machine.vi"("State(s) in (\"\")"="Macro: Initialize") -> ("States Out"=w8:string)  [unwired: 14 in]
  n2 = while "JKI - String-Based Queued State Machine (Basic) v1.0" {
    shift-right: [w14] -> w6
    shift-left: _ -> [w13]
    shift-right: [w17] -> w2
    shift-left: "Error In" -> [w11]
    shift-right: [w16] -> _
    shift-left: w8 -> [w18]
    tunnel: "Lockin" -> [w10]
    tunnel: "KH" -> [w9]
    stop <- w15 stop-if-true
    w12 = -1  # Timeout
    # "Template Copyright © 2015 JKI - http://jki.net/state-machine"
    n3 = call <vilib>:"Parse State Queue__jki_lib_state_machine.vi"("State Queue"=w18, "Error In (no error)"=w11) -> ("Remaining States"=w20:string, "Current State"=w21:string, "Arguments"=w19:string)  [unwired: 11 in]
    n4 = case shown="\"Metadata: Update Control Experiment Wire\"" w21 {
      selector: w21 -> [_ _ w195 _ _ _ _ _ _ _ _ _ _ _ _ _ _ _ _ _ _ _ _ _ _ _ _ _ _ _ _ _ _ _ _ _ _ _ _ _ _ _ _ _ _ _ _ _ _ _ _ _ _ _ _ _]
      tunnel: w20 -> [w28 w194 w199 w217 w223 w228 w232 w253 w264 w279 w315 w323 w327 w346 w378 w387 w398 w424 w439 w452 w456 w461 w472 w479 w492 w497 w502 w506 w518 w534 w560 w574 w583 w596 w603 w629 w633 w651 w684 w771 w786 w794 w805 w822 w837 w841 w849 w867 w898 w914 w935 w949 w954 w958 w968 w986]
      tunnel: w19 -> [_ _ _ _ _ _ _ _ _ _ _ _ _ _ _ w382 w392 _ _ _ _ _ _ _ _ _ _ _ _ _ _ _ _ _ _ _ _ _ _ _ _ _ _ _ _ _ _ _ _ _ _ _ _ _ _ _]
      tunnel: w13 -> [w26 w191 w197 w208 w220 w226 w229 _ w259 w275 w294 w318 w324 w335 w353 w385 w394 w421 w436 w450 w453 w458 w469 w477 w489 w494 w499 w503 w514 w530 w557 w572 w579 w594 w601 w620 w630 w649 w676 w764 w783 w792 w798 w818 w827 w838 w843 w851 w883 w911 w922 w947 w952 w955 w960 w984]
      tunnel: [w25 w192 w201 w214 errorcluster {"status"=FALSE, "code"=0, "source"=""} ("error out") w225 w230 w250 w262 w270 w295 w321 w325 w336 w376 w383 w395 w422 w437 w440 w454 w459 w470 w475 w490 w495 w500 w504 w516 w532 w544 w564 w576 w584 w599 w615 w631 w635 w675 w768 w784 w788 w802 w816 w828 w839 w847 w860 w880 w912 w933 w942 w950 w956 w961 w972] -> w17
      tunnel: w11 -> [w24 w192 w200 w214 w219 w225 w230 w250 w262 w276 w296 w319 w325 w344 w376 w384 w396 w422 w437 w447 w454 w459 w470 w475 w490 w495 w500 w504 w516 w532 w542 w565 w576 w585 w597 w617 w631 w645 w675 w760 w784 w787 w803 w819 w829 w839 w847 w850 w896 w912 w933 w943 w951 w956 w962 w974]
      tunnel: [w27 w193 w198 w216 w222 w227 w231 w252 w263 w278 w314 w322 w326 w345 w377 w386 w397 w423 w438 w451 w455 w460 w471 w478 w491 w496 w501 w505 w517 w533 w559 w573 w582 w595 w602 w628 w632 w650 w683 w770 w785 w793 w804 w821 w836 w840 w848 w866 w897 w913 w934 w948 w953 w957 w967 w985] -> w16
      tunnel: [_ _ _ _ _ TRUE _ _ _ _ _ _ _ _ _ _ _ _ _ _ _ _ _ _ _ _ _ _ _ _ _ _ _ _ _ _ _ _ _ _ _ _ _ _ _ _ _ _ _ _ _ _ _ _ _ _] -> w15
      tunnel: [w23 w191 w197 w215 w220 w226 w229 w251 w258 w274 w285 w318 w324 w335 w353 w385 w394 w421 w436 w450 w453 w458 w469 w477 w489 w494 w499 w503 w515 w531 w558 w571 w578 w593 w601 w620 w630 w648 w682 w769 w783 w791 w797 w817 w835 w838 w842 w861 w883 w911 w921 w947 w952 w955 w959 w984] -> w14
      tunnel: w12 -> [w22 _ _ _ _ _ _ _ _ _ _ _ _ _ _ _ _ _ _ _ _ _ _ _ _ _ _ _ _ _ _ _ _ _ _ _ _ _ _ _ _ _ _ _ _ _ _ _ _ _ _ _ _ _ _ _]
      tunnel: w10 -> [_ _ _ _ _ _ _ w234 _ _ _ _ _ _ _ _ _ _ _ _ _ _ _ _ _ _ _ _ _ _ _ _ _ _ _ _ _ _ _ _ _ _ _ _ _ _ _ _ _ _ _ _ _ _ _ _]
      tunnel: w9 -> [_ _ _ _ _ _ _ w233 _ _ _ _ _ _ _ _ _ _ _ _ _ _ _ _ _ _ _ _ _ _ _ _ _ _ _ _ _ _ _ _ _ _ _ _ _ _ _ _ _ _ _ _ _ _ _ _]
      frame "", "Event Structure", "Idle" {
        # "executes when the state queue is empty"
        n5 = event shown="[17] Panel Close?" {
          selector: _ -> [_ _ _ _ _ _ _ _ _ _ _ _ _ _ _ _ _ _]
          dyn-events: _ -> [_ _ _ _ _ _ _ _ _ _ _ _ _ _ _ _ _ _]
          timeout: w22 -> [_ _ _ _ _ _ _ _ _ _ _ _ _ _ _ _ _ _]
          tunnel: w28 -> [w32 w40 w51 w58 w64 w70 w77 w83 w88 w93 w95 w100 w117 w152 w157 w172 w184 w190]
          tunnel: [w31 w39 w53 w57 w63 w69 w76 w82 w87 w92 w95 w100 w116 w152 w156 w171 w183 w189] -> w27
          tunnel: w26 -> [w29 w37 w52 w55 w61 w67 w75 w81 w86 w91 w94 w99 w115 w153 w158 w170 w181 w187]
          tunnel: [w30 w38 w50 w56 w62 w68 w72 w79 w84 w89 w96 w101 w104 w154 w159 w173 w182 w188] -> w25
          tunnel: w24 -> [w30 w38 w50 w56 w62 w68 w73 w79 w84 w89 w97 w102 w113 w154 w159 w173 w182 w188]
          tunnel: [w29 w37 w52 w55 w61 w67 w75 w81 w86 w91 w94 w99 w115 w153 w158 w170 w181 w187] -> w23
          event Timeout {
            n6 = event-data() -> ()  [unwired: 1 in, 1 out]
            n7 = call <vilib>:"Add State(s) to Queue__jki_lib_state_machine.vi"("State(s) in (\"\")"=w32) -> ("States Out"=w31:string)  [unwired: 14 in]
          }
          event "Krohn Hite?": Value Change {
            # "DONE in new UI"
            n8 = event-data() -> ("NewVal"=w33:bool)  [unwired: 1 in, 5 out]
            n9 = local read "#AI"() -> (w34:u32)
            n10 = case shown="True" w33 {
              tunnel: [w43 w44] -> w35
              tunnel: w34 -> [w42 w45]
              frame False {
                n11 = Initialize Array(T11."none" ("Enum"), w42) -> (w43:T21)
              }
              frame True {
                n12 = for {
                  N: w45 -> [_]
                  tunnel: [w46] -> w44 mode=indexing
                  i -> [w47]
                  n13 = Variant To Data(type=T11."A 1" ("Enum"), Variant=w47) -> (data=w46:T11)  [unwired: 1 in, 1 out]
                }
              }
            }
            n14 = control-ref of="KH #"() -> (w36:refnum<vi>)
            n15 = property on="KH Addresses" class="Arr (strict)"("Visible"=w33) -> ()  [unwired: 2 in, 2 out]
            n16 = property class="Arr (strict)"(reference=w36, "Value"=w35) -> ()  [unwired: 1 in, 2 out]
            n17 = call <vilib>:"Add State(s) to Queue__jki_lib_state_machine.vi"("State(s) in (\"\")"=w40) -> ("States Out"=w39:string)  [unwired: 14 in]
          }
          event "Labels Strings": Value Change {
            # "DONE in new UI"
            n18 = event-data() -> ()  [unwired: 1 in, 6 out]
            n19 = property on="Ring" class="Ring (strict)"("Strings []"="Labels Strings") -> ()  [unwired: 2 in, 2 out]
            n20 = property on="Ring" class="Ring (strict)"("Strings []"="Labels Strings") -> ()  [unwired: 2 in, 2 out]
            n21 = call <vilib>:"Add State(s) to Queue__jki_lib_state_machine.vi"("State(s) in (\"\")"=w51) -> ("States Out"=w53:string)  [unwired: 14 in]
          }
          event "OK": Value Change {
            # "DONE in new UI"
            # "Exit Button Value Change (pressed) Event\n(this executes Macro: Exit to terminate the VI)"
            n22 = event-data() -> ()  [unwired: 1 in, 1 out]
            n23 = call <vilib>:"Add State(s) to Queue__jki_lib_state_machine.vi"("State(s) in Front (\"\")"="Macro: Exit", "State(s) in (\"\")"=w58) -> ("States Out"=w57:string)  [unwired: 13 in]
          }
          event "Open VI": Value Change {
            # "DONE in new UI"
            # "Exit Button Value Change (pressed) Event\n(this executes Macro: Exit to terminate the VI)"
            n24 = event-data() -> ()  [unwired: 1 in, 6 out]
            n25 = local write "Open VI"(FALSE ("Open VI")) -> ()
            n26 = call <vilib>:"Add State(s) to Queue__jki_lib_state_machine.vi"("State(s) in Front (\"\")"="Experiment VI: Open VI", "State(s) in (\"\")"=w64) -> ("States Out"=w63:string)  [unwired: 13 in]
          }
          event "Open Lockin": Value Change {
            # "DONE in new UI"
            # "Exit Button Value Change (pressed) Event\n(this executes Macro: Exit to terminate the VI)"
            n27 = event-data() -> ()  [unwired: 1 in, 6 out]
            n28 = local write "Open Lockin"(FALSE ("Open VI")) -> ()
            n29 = call <vilib>:"Add State(s) to Queue__jki_lib_state_machine.vi"("State(s) in Front (\"\")"="Experiment VI: Open Lockin", "State(s) in (\"\")"=w70) -> ("States Out"=w69:string)  [unwired: 13 in]
          }
          event "Create Output": Value Change {
            # "#todo in new UI"
            # "\"Create Output\" Value Change (pressed) Event\n(this executes Macro: Output)"
            n30 = event-data() -> ()  [unwired: 1 in, 6 out]
            n31 = invoke on="Create Output" class="Bool" method="Reinit To Default"(error in=w73) -> (error out=w72:errorcluster)  [unwired: 2 in, 2 out]
            n32 = property on="Values have changed" class="Bool (strict)"("Val(Sgnl)"=FALSE ("Value (Signaling)")) -> ()  [unwired: 2 in, 2 out]
            n33 = call <vilib>:"Add State(s) to Queue__jki_lib_state_machine.vi"("State(s) in Front (\"\")"="Macro: Output", "State(s) in (\"\")"=w77) -> ("States Out"=w76:string)  [unwired: 13 in]
          }
          event "Values have changed": Value Change {
            # "#todo in new UI"
            # "\"Values have changed\" Value Change (pressed) Event\n(this executes Macro: Output)"
            n34 = event-data() -> ("NewVal"=w78:bool)  [unwired: 1 in, 5 out]
            n35 = property on="Values have changed" class="Bool (strict)"("Blinking"=w78) -> ()  [unwired: 2 in, 2 out]
            n36 = property on="String" class="Str"("Blinking"=w78) -> ()  [unwired: 2 in, 2 out]
            n37 = call <vilib>:"Add State(s) to Queue__jki_lib_state_machine.vi"("State(s) in Front (\"\")"="", "State(s) in (\"\")"=w83) -> ("States Out"=w82:string)  [unwired: 13 in]
          }
          event "Write Pickering Config": Value Change {
            # "DON't"
            # "\"Create Output\" Value Change (pressed) Event\n(this executes Macro: Output)"
            n38 = event-data() -> ()  [unwired: 1 in, 6 out]
            n39 = call <vilib>:"Add State(s) to Queue__jki_lib_state_machine.vi"("State(s) in Front (\"\")"="", "State(s) in (\"\")"=w88) -> ("States Out"=w87:string)  [unwired: 13 in]
          }
          event "Read Pickering Config": Value Change {
            # "DON't"
            # "\"Create Output\" Value Change (pressed) Event\n(this executes Macro: Output)"
            n40 = event-data() -> ()  [unwired: 1 in, 6 out]
            n41 = call <vilib>:"Add State(s) to Queue__jki_lib_state_machine.vi"("State(s) in Front (\"\")"="", "State(s) in (\"\")"=w93) -> ("States Out"=w92:string)  [unwired: 13 in]
          }
          event "C Bridge?": Value Change {
            # "DONE in new UI"
            n42 = event-data() -> ("NewVal"=w98:bool)  [unwired: 1 in, 5 out]
            n43 = property on="Capacitance Bridge Address" class="VISAName"(error in=w97, "Visible"=w98) -> (error out=w96:errorcluster)  [unwired: 1 in, 1 out]
          }
          event "Strain Cell?": Value Change {
            # "DONE"
            n44 = event-data() -> ("NewVal"=w103:bool)  [unwired: 1 in, 5 out]
            n45 = property on="Strain Cell Address" class="VISAName"(error in=w102, "Visible"=w103) -> (error out=w101:errorcluster)  [unwired: 1 in, 1 out]
          }
          event "Lockin.Label": Value Change {
            # "DONE"
            # "F: not found\nground\nT: found:\n0 - Vsg - gate\n1 - Vbg - gate\n2 - I ----- current\n????:\n4 - V ---- voltage\n3 - dV(?) voltage diff"
            # "Label Value Change Event\n(chooses proper configuration for amplifiers)"
            n46 = event-data() -> ("NewVal"=w114:u16[])  [unwired: 1 in, 5 out]
            n47 = for {
              tunnel: w114 -> [w125] mode=indexing
              tunnel: [w127] -> w109 mode=indexing
              tunnel: w113 -> [w124]
              tunnel: [w123] -> w104
              tunnel: [w122] -> w106 mode=indexing
              tunnel: [w118] -> w107 mode=indexing
              n48 = property on="Label" class="Ring (strict)"(error in=w124) -> (error out=w123:errorcluster, "Strings []"=w126:string[])  [unwired: 1 in, 1 out]
              n49 = Index Array(array=w126, index=w125) -> (element=w121:string)
              n50 = call <userlib>:"MGI String Pattern Match Exists.vi"("Patterns to Try"=string[] ["Vsg", "Vbg", "I", "dV", "V"], "String"=w121) -> ("Index of First Pattern Matched"=w128:i32, "Match Found"=w119:bool)
              n51 = case shown="True" w119 {
                tunnel: w128 -> [_ w135]
                tunnel: [KH_Mode-enum."Ground" ("Enum") w134] -> w127
                tunnel: [Shunt-Enum."Open" ("Shunt Resistor") w133] -> w122
                tunnel: [Input_Configuration-Enum."Ground" ("Input Configuation") w132] -> w118
                frame False {
                }
                frame True {
                  n52 = case shown="0, Default" w135 {
                    tunnel: [KH_Mode-enum."Gate" ("Enum") KH_Mode-enum."Gate" ("Enum") KH_Mode-enum."Current" ("Enum") KH_Mode-enum."Voltage (Diff)" ("Enum") KH_Mode-enum."Voltage (SE)" ("Enum")] -> w134
                    tunnel: [Shunt-Enum."50k Ohms" ("Shunt Resistor") Shunt-Enum."50k Ohms" ("Shunt Resistor") "Defualt Shunt Resistor" Shunt-Enum."Open" ("Shunt Resistor") Shunt-Enum."Open" ("Shunt Resistor")] -> w133
                    tunnel: [Input_Configuration-Enum."Differential" ("Input Configuation") Input_Configuration-Enum."Differential" ("Input Configuation") Input_Configuration-Enum."Differential" ("Input Configuation") Input_Configuration-Enum."Differential" ("Input Configuation") Input_Configuration-Enum."SE+ (-gnd)" ("Input Configuation")] -> w132
                    frame 0, Default {
                      # "Vsg - gate"
                    }
                    frame 1 {
                      # "Vbg - gate"
                    }
                    frame 2 {
                      # "I - current"
                    }
                    frame 3 {
                      # "dV - V (Diff)"
                    }
                    frame 4 {
                      # "V - V (SE)"
                    }
                  }
                }
              }
            }
            n53 = property on="Values have changed" class="Bool (strict)"("Val(Sgnl)"=FALSE ("Values have changed")) -> ()  [unwired: 2 in, 2 out]
            n54 = local read "Lockin"() -> (w111:T7)
            n55 = Bundle By Name(cluster=w111, "Electrode Config"=w109) -> (w110:T7)
            n56 = local read "KH"() -> (w108:T5)
            n57 = Bundle By Name(cluster=w108, "KH Shunt Resistor"=w106, "KH Configuration"=w107) -> (w105:T5)
            n58 = local write "Lockin"(w110) -> ()
            n59 = local write "KH"(w105) -> ()
            n60 = call <vilib>:"Add State(s) to Queue__jki_lib_state_machine.vi"("State(s) in (\"\")"=w117) -> ("States Out"=w116:string)  [unwired: 14 in]
          }
          event "KH.KH Shunt Resistor", "KH.KH Gain", "non KH.Electrodes 2", "non KH.Labels 2", "Sample (SAXXXX)", "Username", "Description", "Lockin.Electrode": Value Change {
            # "#todo"
            n61 = event-data() -> ()  [unwired: 1 in, 6 out]
            n62 = property on="Values have changed" class="Bool (strict)"("Val(Sgnl)"=TRUE ("Values have changed")) -> ()  [unwired: 2 in, 2 out]
          }
          event "Lockin.AI", "non KH.Scroll Bar": Mouse Move; "Lockin.AI", "non KH.Scroll Bar": Mouse Wheel {
            # "DON't"
            n63 = event-data() -> ()  [unwired: 1 in, 5 out]
            n64 = call <vilib>:"Add State(s) to Queue__jki_lib_state_machine.vi"("State(s) in Front (\"\")"="UI: Link Scroll Bars" ("State(s) in Front (\"\")"), "State(s) in (\"\")"=w157) -> ("States Out"=w156:string)  [unwired: 13 in]
          }
          event "#AI": Value Change {
            # "DONE (I think)"
            n65 = event-data() -> ("NewVal"=w166:u32)  [unwired: 1 in, 5 out]
            n66 = for {
              N: w166 -> [_]
              tunnel: [w175] -> w160 mode=indexing
              tunnel: [w174] -> w161 mode=indexing
              i -> [w174]
              n67 = Increment(x=w174) -> (x+1=w175:i32)
            }
            n68 = local read "Lockin"() -> (w169:T7)
            n69 = Bundle By Name(cluster=w169, "AI"=w160) -> (w168:T7)
            n70 = local write "Lockin"(w168) -> ()
            n71 = Initialize Array(1.0 ("element"), w166) -> (w164:dbl[])
            n72 = local read "KH"() -> (w163:T5)
            n73 = local write "Gain"(w164) -> ()
            n74 = Bundle By Name(cluster=w163, "KH #"=w161) -> (w167:T5)
            n75 = local write "KH"(w167) -> ()
            n76 = call <vilib>:"Add State(s) to Queue__jki_lib_state_machine.vi"("State(s) in Front (\"\")"="Metadata: Update KH\nKH: set KH 0\nKH: set KH 1" ("State(s) in Front (\"\")"), "State(s) in (\"\")"=w172) -> ("States Out"=w171:string)  [unwired: 13 in]
          }
          event "KH Addresses": Value Change {
            n77 = event-data() -> ()  [unwired: 1 in, 6 out]
            n78 = local read "KH"() -> (w176:T5)
            n79 = Unbundle By Name(w176) -> ("KH #"=w178:u16[])
            n80 = Array Subset(array=w178) -> (w177:u16[])  [unwired: 2 in]
            n81 = Bundle By Name(cluster=w176, "KH #"=w177) -> (w179:T5)
            n82 = local write "KH"(w179) -> ()
            n83 = call <vilib>:"Add State(s) to Queue__jki_lib_state_machine.vi"("State(s) in Front (\"\")"="KH: set KH 0\nKH: set KH 1", "State(s) in (\"\")"=w184) -> ("States Out"=w183:string)  [unwired: 13 in]
          }
          event Panel Close? {
            # "Discard the event because we'll close the front panel ourselves in Macro: Exit"
            # "Close Panel button (pressed) Event\n(this executes Macro: Exit to terminate the VI)"
            n84 = event-data() -> ()  [unwired: 1 in, 1 out]
            n85 = event-data("Discard?"=TRUE) -> ()  [unwired: 1 in, 1 out]
            n86 = call <vilib>:"Add State(s) to Queue__jki_lib_state_machine.vi"("State(s) in Front (\"\")"="Macro: Exit", "State(s) in (\"\")"=w190) -> ("States Out"=w189:string)  [unwired: 13 in]
          }
        }
      }
      frame "---------- Core ----------" {
        # "Do not put any code in this frame.\n(it is a separator no-op)"
        n87 = call <vilib>:"Add State(s) to Queue__jki_lib_state_machine.vi"("State(s) in (\"\")"=w194) -> ("States Out"=w193:string)  [unwired: 14 in]
      }
      frame Default {
        w204 = 42 items=["No error", "Argument error", "Memory is full", "Out of zone", "End of file", "File already open", "Generic file I/O error", "File not found", "File permission error", "Disk is full", "Duplicate path", "Too many files open", "System feature not enabled", "Resource file not found", "Cannot add resource", "Resource not found", "Image not found", "Image memory error", "Pen does not exist", "Config type invalid", "Config token not found", "Config parse error", "Config memory error", "Bad external code format", "Bad external code offset", "External code not present", "Null window", "Destroy window error", "Null menu", "Print aborted", "Bad print record", "Print driver error", "Windows error during printing", "Memory error during printing", "Print dialog error", "Generic print error", "Invalid device refnum", "Device not found", "Device parameter error", "Device unit error", "Cannot open device", "Device call aborted", "Generic error", "Cancelled by user", "Object ID too low", "Object ID too high", "Object not in heap", "Unknown heap", "Unknown object (invalid DefProc)", "Unknown object (DefProc not in table)", "Message out of range", "Invalid (null) method", "Unknown message", "Manager call not supported", "Bad address", "Network operation in progress", "Network operation timed out", "Connection is busy", "Network attribute not supported", "Network error", "Address in use", "System out of memory", "Connection aborted", "Connection refused", "Not connected", "Already connected", "Connection closed", "Initialization error (interapplication manager)", "Bad occurrence", "Wait on unbound occurrence handler", "Occurrence queue overflow", "Datalog type conflict", "Unused", "Unrecognized type (interapplication manager)", "Memory corrupt", "Failed to make temporary DLL", "Old CIN version", "Drag socket not found", "Failed to load drop-object", "Failed to register OLE object", "Failed to release OLE object", "Format specifier type mismatch", "Unknown format specifier", "Too few format specifiers", "Too many format specifiers", "Scan failed", "Newer CIN version", "Error converting to variant", "Runtime menu error", "Password tampered", "Variant attribute not found", "Incompatible variant data type", "Event data is not available", "Event Store is not present", "Occurrence is not found", "Event Queue is not created", "Event info is not available", "Refnum passed is NULL", "Error retrieving Class GUID", "Error retrieving CoClass GUID", "Error retrieving TypeLib GUID.", "Bad built application magic bytes.", "Specific driver is different from the specific driver associated with the Logical Name.", "There is no session opened to the class driver.", "Max Error", "MAX - Error with config objects", "MAX - Error loading configuration", "MAX - Group not supported"]
        # "Current State"
        # "Do not delete, rename, or modify this frame.\n(this is used to capture unhandled states and typos)"
        # "Handle mistyped state name (developer tool)"
        n88 = Format Into String(format string="Software Exception: Unhandled State \"%s\"." ("message"), error in=w200, w195) -> (resulting string=w203:string, error out=w202:errorcluster)  [unwired: 1 in]
        n89 = call <vilib>:"Error Cluster From Error Code.vi"("show call chain? (False)"=TRUE, "error in (no error)"=w202, "error message (\"\")"=w203, "error code (0)"=w204) -> ("error out"=w201:errorcluster)  [unwired: 5 in]
        n90 = call <vilib>:"Add State(s) to Queue__jki_lib_state_machine.vi"("State(s) in (\"\")"=w199) -> ("States Out"=w198:string)  [unwired: 14 in]
      }
      frame "Initialize Core Data" {
        # "Do not delete, rename, or modify this frame.\n(this is used to determine panel behavior on exit)"
        # "originally closed?"
        # "exe?"
        # "If panel starts closed or is an EXE, then close it when we exit"
        n91 = property class="VI"() -> ("Front Panel.Open"=w213:bool)  [unwired: 2 in, 2 out]
        n92 = property class="App"() -> ("App.Kind"=w212:T12)  [unwired: 2 in, 2 out]
        n93 = control-ref of="Current VI Reference"() -> (w206:refnum<vi>)
        n94 = Not(x=w213) -> (.not. x?=w210:bool)
        n95 = Equal?(x=w212, y=T12."Run Time System" ("Application:Kind")) -> (x = y?=w209:bool)
        n96 = Or(x=w210, y=w209) -> (x .or. y?=w207:bool)
        n97 = Bundle By Name(cluster=w208, "Core.Current VI Reference"=w206, "Core.Close Panel on Exit?"=w207) -> (w215:T27)
        n98 = call <vilib>:"Add State(s) to Queue__jki_lib_state_machine.vi"("State(s) in (\"\")"=w217) -> ("States Out"=w216:string)  [unwired: 14 in]
      }
      frame "Error Handler" {
        # "Unhandled Error -- Display it"
        # "Handle any errors here.\nYou can also output any states to clean-up after errors occur"
        # "Clear error"
        n99 = call <vilib>:"General Error Handler.vi"("error in (no error)"=w219) -> ()  [unwired: 10 in, 5 out]
        n100 = call <vilib>:"Add State(s) to Queue__jki_lib_state_machine.vi"("State(s) in Front (\"\")"="/* Post Error States", "State(s) in (\"\")"=w223) -> ("States Out"=w222:string)  [unwired: 13 in]
      }
      frame "Exit" {
        # "Do not put any code in this frame.\n(No errors that occur here will be handled.)"
        n101 = call <vilib>:"Add State(s) to Queue__jki_lib_state_machine.vi"("State(s) in (\"\")"=w228) -> ("States Out"=w227:string)  [unwired: 14 in]
      }
      frame "---------- Data ----------" {
        # "Do not put any code in this frame.\n(It is a separator no-op. You can make a copy of this frame to create a new Data frame)"
        n102 = call <vilib>:"Add State(s) to Queue__jki_lib_state_machine.vi"("State(s) in (\"\")"=w232) -> ("States Out"=w231:string)  [unwired: 14 in]
      }
      frame "Data: Initialize" {
        w235 = TRUE  # top level?
        w236 = path[] []  # VI paths
        w237 = refnum<class "Logger.PGSQL.lvclass"> refnum  # Logger
        w238 = T25 {"Sample"="", "Device"="", "Username"="", "Description"="", "Default Path"=path "", "AWS Path"=path "", "Instrument"=enum."----- AFM/EBL -----", "Lockin?"=FALSE, "Lockin Address"="", "Krohn Hite?"=FALSE, "KH Addresses"=[], "KH All Buttons"=enum."No Selection", "Strain Cell?"=FALSE, "Strain Cell Address"="", "C Bridge?"=FALSE, "Capacitance Bridge Address"="", "Lockin"={"AI"=[], "Electrode"=[], "Label"=[], "Electrode Config"=[]}, "KH"={"KH #"=[], "KH Configuration"=[], "KH Gain"=[], "KH Shunt Resistor"=[], "Filter"=FALSE, "DC Coupled"=FALSE}, "non KH"={"Scroll Bar"=[], "Electrodes 2"=[], "Labels 2"=[], "unused"=[]}, "#AI"=8}  # UI
        w242 = refnum<class "Configuration.lvclass"> refnum  # Config
        w246 = T28 {"Authentication Info"={"Client ID"="1150712142949183", "Client Secret"="530770942aed47201cd52aeb331bdd57", "Redirect URI"="https://www.google.com/", "Token Endpoint"="https://app.asana.com/-/oauth_token", "Scope"=""}, "Authentication Header"=[], "Refresh Token"="", "Time Stamp"=timestamp(0 s since 1904-01-01)}  # Asana
        w247 = cluster{"Channel Setting":T24}[] []  # Channel Settings
        w240 = T29 {"Current VI Reference"=refnum, "Close Panel on Exit?"=FALSE}  # Core
        # "Initialize the shift-register data, here.\n(data names are defined by what you wire into the bundle function)"
        n103 = local read "Refresh Token Out"() -> (w245:string)
        n104 = Unbundle By Name("C.E.") -> ("Experiment"=w248:T22, "Wiring"=w249:T23)
        n105 = Bundle By Name(cluster=w246, "Refresh Token"=w245) -> (w244:T28)
        n106 = Bundle("Core"=w240, "C.E."="C.E.", "Experiment"=w248, "Wiring"=w249, "Channel Settings"=w247, "KH All Buttons"="KH All Buttons", "Lockin"=w234, "KH"=w233, "non KH"="non KH", "UI"=w238, "Asana"=w244, "Logger"=w237, "Config"=w242, "VI paths"=w236, "top level?"=w235) -> (w251:T27)  [unwired: 1 in]
        n107 = call <vilib>:"Add State(s) to Queue__jki_lib_state_machine.vi"("State(s) in (\"\")"=w253) -> ("States Out"=w252:string)  [unwired: 14 in]
      }
      frame "Data: Initialize Top Level" {
        # "Do not put any code in this frame.\n(It is a separator no-op. You can make a copy of this frame to create a new Data frame)"
        n108 = property class="VI"() -> ("Exec.State"=w261:T13)  [unwired: 2 in, 2 out]
        n109 = Equal?(x=w261, y=T13."Run top level" ("Execution:State")) -> (x = y?=w257:bool)
        n110 = Select(t="", s=w257, f="Macro: Output\nMacro: Exit") -> (s? t:f=w256:string)
        n111 = Bundle By Name(cluster=w259, "top level?"=w257) -> (w258:T27)
        n112 = call <vilib>:"Add State(s) to Queue__jki_lib_state_machine.vi"("State(s) in (\"\")"=w264, "State(s) at Back (\"\")"=w256) -> ("States Out"=w263:string)  [unwired: 13 in]
      }
      frame "Data: Load Configuration" {
        # "DONE"
        n113 = disable-structure shown="Disabled" {
          frame Disabled {
            w283 = T30 7 items=["User Home"=0, "User Desktop"=1, "User Documents"=2, "User Application Data"=3, "User Preferences"=4, "User Temporary"=5, "Public Documents"=6, "Public Application Data"=7, "Public Preferences"=8, "Public Cache"=13, "System Core Libraries"=9, "System Installed Libraries"=10, "Application Files"=11, "Boot Volume Root"=12] ("system directory type")
            n114 = call <vilib>:"Get System Directory.vi"("system directory type"=w283) -> ("system directory"=w280:path)  [unwired: 10 in]
            n115 = Build Path(base path=w280, name or relative path="Levylab") -> (appended path=w282:path)
            n116 = Build Path(base path=w282, name or relative path="Control Experiment") -> ()  [unwired: 1 out]
          }
          frame Enabled {
          }
        }
        n117 = Unbundle By Name(w275) -> ("Config"=w277:refnum<class "Configuration.lvclass">, "UI"=w269:T25)
        n118 = call <userlib>:"Current VIs Parent Directory__ogtk.vi"() -> ("Parent Directory (+ Relative)"=w265:path)  [unwired: 5 in]
        n119 = call <userlib>:"Write Path.vi"("error in (no error)"=w276, "Path"=w265, "Configuration in"=w277) -> ("error out"=w272:errorcluster, "Configuration out"=w273:refnum<class "Configuration.lvclass">)  [unwired: 7 in]
        n120 = call <userlib>:"Read Configuration.vi"("INI Fomatted Cluster Type"=w269, "error in (no error)"=w272, "Configuration in"=w273) -> ("error out"=w271:errorcluster, "Configuration"=w267:variant, "Configuration out"=w268:refnum<class "Configuration.lvclass">)  [unwired: 6 in]
        n121 = Variant To Data(error in=w271, type=w269, Variant=w267) -> (data=w266:T25, error out=w270:errorcluster)
        n122 = Bundle By Name(cluster=w275, "Config"=w268, "UI"=w266) -> (w274:T27)
        n123 = call <vilib>:"Add State(s) to Queue__jki_lib_state_machine.vi"("State(s) in (\"\")"=w279) -> ("States Out"=w278:string)  [unwired: 14 in]
      }
      frame "Data: Save Controls" {
        # "DONE"
        n124 = local read "Sample (SAXXXX)"() -> (w313:string)
        n125 = local read "Username"() -> (w311:string)
        n126 = local read "Default Path"() -> (w309:path)
        n127 = local read "Strain Cell?"() -> (w303:bool)
        n128 = local read "C Bridge?"() -> (w301:bool)
        n129 = local read "Lockin"() -> (w299:T7)
        n130 = local read "Lockin Address"() -> (w307:string)
        n131 = local read "KH Addresses"() -> (w305:refnum<visa-resource-name>[])
        n132 = local read "KH"() -> (w292:T5)
        n133 = local read "Description"() -> (w310:string)
        n134 = local read "Strain Cell Address"() -> (w302:refnum<visa-resource-name>)
        n135 = local read "Capacitance Bridge Address"() -> (w300:refnum<visa-resource-name>)
        n136 = local read "Instrument"() -> (w308:T9)
        n137 = local read "Device (YYYYMMDD)"() -> (w312:string)
        n138 = Unbundle By Name(w292) -> ("KH #"=w291:u16[], "KH Configuration"=w288:T2[], "KH Gain"=w289:T3[], "KH Shunt Resistor"=w290:T4[])
        n139 = local read "Krohn Hite?"() -> (w306:bool)
        n140 = local read "KH All Buttons"() -> (w304:T8)
        n141 = local read "non KH"() -> (w293:T10)
        n142 = Bundle By Name(cluster=w294, "UI.Sample"=w313, "Experiment.Device"=w312, "UI.Username"=w311, "UI.Description"=w310, "UI.Default Path"=w309, "Experiment.Instrument"=w308, "UI.Lockin Address"=w307, "UI.Krohn Hite?"=w306, "UI.KH Addresses"=w305, "KH All Buttons"=w304, "UI.Strain Cell?"=w303, "UI.Strain Cell Address"=w302, "UI.C Bridge?"=w301, "UI.Capacitance Bridge Address"=w300, "Lockin"=w299, "non KH"=w293, "KH.KH #"=w291, "KH.KH Configuration"=w288, "KH.KH Gain"=w289, "KH.KH Shunt Resistor"=w290, "UI.KH.Filter"="Bandwidth Filter", "UI.KH.DC Coupled"="DC Coupled") -> (w285:T27)
        n143 = Unbundle By Name(w285) -> ("Config"=w298:refnum<class "Configuration.lvclass">, "UI"=w297:T25)
        n144 = call <userlib>:"Write Configuration.vi"("error in (no error)"=w296, "Variant"=w297, "Configuration in"=w298) -> ("error out"=w295:errorcluster)  [unwired: 7 in, 1 out]
        n145 = call <vilib>:"Add State(s) to Queue__jki_lib_state_machine.vi"("State(s) in (\"\")"=w315) -> ("States Out"=w314:string)  [unwired: 14 in]
      }
      frame "Data: Cleanup" {
        # "Cleanup any data and references, here.\n(this is called automatically, by the Macro: Exit)"
        n146 = Unbundle By Name(w318) -> ("Core.Current VI Reference"=w317:refnum<vi>, "Logger"=w320:refnum<class "Logger.PGSQL.lvclass">)
        n147 = call <vilib>:"Stop.vi"("error in (no error)"=w319, "SMO"=w320) -> ("error out"=w316:errorcluster)  [unwired: 8 in, 1 out]
        n148 = Close Reference(reference=w317, error in (no error)=w316) -> (error out=w321:errorcluster)
        n149 = call <vilib>:"Add State(s) to Queue__jki_lib_state_machine.vi"("State(s) in (\"\")"=w323) -> ("States Out"=w322:string)  [unwired: 14 in]
      }
      frame "---------- UI ----------" {
        # "Do not put any code in this frame.\n(It is a separator no-op. You can make a copy of this frame to create a new UI frame)"
        n150 = call <vilib>:"Add State(s) to Queue__jki_lib_state_machine.vi"("State(s) in (\"\")"=w327) -> ("States Out"=w326:string)  [unwired: 14 in]
      }
      frame "UI: Initialize" {
        w330 = TRUE ("Visible")
        (unwired) string[] ["", "I+", "I-", "V1+", "V1-", "V2+", "V2-", "V3+", "V3-", "V4+", "V4-", "dV1", "dV2", "dV3", "Vsg", "Vbg"] ("Strings [] 2")
        # "DONE"
        # "Pickering? = False always"
        # "Initialize the User Interface, here.\n(this is called automatically, by the Macro: Init)"
        n151 = local read "Labels Strings"() -> (w339:string[])
        n152 = call <userlib>:"Fit VI window to Largest Dec__ogtk.vi"("error in (no error)"=w344) -> ("error out"=w341:errorcluster)  [unwired: 5 in, 1 out]
        n153 = Unbundle By Name(w335) -> ("UI.Krohn Hite?"=w333:bool, "UI.Strain Cell?"=w332:bool, "UI.C Bridge?"=w331:bool, "top level?"=w328:bool)
        n154 = property on="OK" class="Bool (strict)"("Value"=FALSE ("Blinking")) -> ()  [unwired: 2 in, 2 out]
        n155 = property on="Ring" class="Ring (strict)"(error in=w341, "Strings []"=w339) -> (error out=w340:errorcluster)  [unwired: 1 in, 1 out]
        n156 = local write "KH All Buttons"(T8."No Selection" ("KH All Buttons")) -> ()
        n157 = property on="Tab Control" class="TabCtl (strict)"("Value"=T1."Input" ("Tab Control")) -> ()  [unwired: 2 in, 2 out]
        n158 = property on="Values have changed" class="Bool (strict)"("Val(Sgnl)"=TRUE ("Blinking")) -> ()  [unwired: 2 in, 2 out]
        n159 = property on="Ring" class="Ring (strict)"(error in=w340, "Strings []"=w339) -> (error out=w342:errorcluster)  [unwired: 1 in, 1 out]
        n160 = property on="Krohn Hite?" class="Bool (strict)"("Val(Sgnl)"=w333, "Visible"=w330) -> ()  [unwired: 2 in, 2 out]
        n161 = disable-structure shown="Enabled" {
          disable-tunnel: w342 -> [_ w349]
          disable-tunnel: [_ w349] -> w336
          disable-tunnel: FALSE ("Blinking") -> [_ _]
          frame Disabled {
          }
          frame Enabled {
          }
        }
        n162 = property on="Strain Cell?" class="Bool (strict)"("Val(Sgnl)"=w332, "Visible"=w330) -> ()  [unwired: 2 in, 2 out]
        n163 = property on="C Bridge?" class="Bool (strict)"("Val(Sgnl)"=w331, "Visible"=w330) -> ()  [unwired: 2 in, 2 out]
        n164 = case shown="True" w328 {
          frame False {
          }
          frame True {
            # "unused"
            n165 = local read "KH Addresses"() -> (w347:refnum<visa-resource-name>[])
            n166 = property on="#AI" class="DigNum (strict)"("Val(Sgnl)"="#AI") -> ()  [unwired: 2 in, 2 out]
            n167 = property on="KH Addresses" class="Arr (strict)"("Val(Sgnl)"=w347) -> ()  [unwired: 2 in, 2 out]
          }
        }
        n168 = call <vilib>:"Add State(s) to Queue__jki_lib_state_machine.vi"("State(s) in (\"\")"=w346) -> ("States Out"=w345:string)  [unwired: 14 in]
      }
      frame "UI: Update Controls" {
        # "DONE"
        # "Do not put any code in this frame.\n(It is a separator no-op. You can make a copy of this frame to create a new Data frame)"
        n169 = Unbundle By Name(w353) -> ("top level?"=w350:bool, "UI.Sample"=w367:string, "UI.Device"=w368:string, "UI.Username"=w369:string, "UI.Description"=w370:string, "UI.Default Path"=w375:path, "UI.Instrument"=w371:T9, "UI.Lockin Address"=w365:string, "UI.Krohn Hite?"=w374:bool, "UI.KH Addresses"=w366:refnum<visa-resource-name>[], "UI.KH All Buttons"=w362:T8, "UI.Strain Cell?"=w373:bool, "UI.Strain Cell Address"=w363:refnum<visa-resource-name>, "UI.C Bridge?"=w372:bool, "UI.Capacitance Bridge Address"=w364:refnum<visa-resource-name>, "UI.Lockin"=w352:T7, "UI.non KH"=w351:T10, "UI.KH.Filter"=w360:bool, "UI.KH.DC Coupled"=w361:bool, "UI.KH.KH #"=w357:T21, "UI.KH.KH Configuration"=w356:T2[], "UI.KH.KH Gain"=w355:T3[], "UI.KH.KH Shunt Resistor"=w354:T4[])
        n170 = local write "Sample (SAXXXX)"(w367) -> ()
        n171 = local write "Krohn Hite?"(w374) -> ()
        n172 = local write "Bandwidth Filter"(w360) -> ()
        n173 = local write "Strain Cell?"(w373) -> ()
        n174 = local write "C Bridge?"(w372) -> ()
        n175 = local write "Username"(w369) -> ()
        n176 = local write "Instrument"(w371) -> ()
        n177 = local write "Default Path"(w375) -> ()
        n178 = local write "KH Addresses"(w366) -> ()
        n179 = local write "Strain Cell Address"(w363) -> ()
        n180 = local write "Capacitance Bridge Address"(w364) -> ()
        n181 = local write "DC Coupled"(w361) -> ()
        n182 = local write "Device (YYYYMMDD)"(w368) -> ()
        n183 = local write "Description"(w370) -> ()
        n184 = local write "Lockin Address"(w365) -> ()
        n185 = local write "KH All Buttons"(w362) -> ()
        n186 = local read "KH"() -> (w359:T5)
        n187 = Bundle By Name(cluster=w359, "KH #"=w357, "KH Configuration"=w356, "KH Gain"=w355, "KH Shunt Resistor"=w354) -> (w358:T5)
        n188 = case shown="True" w350 {
          tunnel: w358 -> [_ w381]
          tunnel: w352 -> [_ w380]
          tunnel: w351 -> [_ w379]
          frame False {
          }
          frame True {
            n189 = local write "non KH"(w379) -> ()
            n190 = local write "Lockin"(w380) -> ()
            n191 = local write "KH"(w381) -> ()
          }
        }
        n192 = call <vilib>:"Add State(s) to Queue__jki_lib_state_machine.vi"("State(s) in (\"\")"=w378) -> ("States Out"=w377:string)  [unwired: 14 in]
      }
      frame "UI: Cursor Set" {
        # "Argument"
        # "Set and Unset Cursor Busy.\n(Usage: \"UI: Cursor Set >> Busy|Idle\")"
        n193 = case shown="\"Busy\"" w382 {
          tunnel: w384 -> [w389 w391]
          tunnel: [w388 w390] -> w383
          frame "Idle", Default {
            n194 = call <vilib>:"Unset Busy.vi"("error in (no error)"=w389) -> ("error out"=w388:errorcluster)  [unwired: 10 in]
          }
          frame "Busy" {
            n195 = call <vilib>:"Set Busy.vi"("error in (no error)"=w391) -> ("error out"=w390:errorcluster)  [unwired: 9 in, 1 out]
          }
        }
        n196 = call <vilib>:"Add State(s) to Queue__jki_lib_state_machine.vi"("State(s) in (\"\")"=w387) -> ("States Out"=w386:string)  [unwired: 14 in]
      }
      frame "UI: Front Panel State" {
        # "Argument"
        # "Set Front Panel Open or Closed\n(Usage: \"UI: Front Panel State >> Open|Close\")"
        n197 = Unbundle By Name(w394) -> ("Core.Current VI Reference"=w393:refnum<vi>)
        n198 = case shown="\"Open\", Default" w392 {
          tunnel: w396 -> [w402 w415]
          tunnel: [w404 w416] -> w395
          tunnel: w393 -> [w403 w413]
          frame "Open", Default {
            n199 = property class="VI"(reference=w403, error in=w402) -> (reference out=w400:refnum<vi>, error out=w401:errorcluster, "Front Panel.Open"=w399:bool)
            n200 = case shown="True" w399 {
              tunnel: [w407 w410] -> w404
              tunnel: w401 -> [w406 w410]
              tunnel: w400 -> [w405 _]
              frame False {
                n201 = invoke class="VI" method="FP.Open"(reference=w405, error in=w406, "Activate"=TRUE, "State"=T14."Standard") -> (error out=w407:errorcluster)  [unwired: 1 in, 4 out]
              }
              frame True {
              }
            }
          }
          frame "Close" {
            n202 = property class="VI"(reference=w413, error in=w415) -> (reference out=w412:refnum<vi>, error out=w414:errorcluster, "Front Panel.Open"=w411:bool)
            n203 = case shown="True" w411 {
              tunnel: [w417 w420] -> w416
              tunnel: w414 -> [w417 w419]
              tunnel: w412 -> [_ w418]
              frame False {
              }
              frame True {
                n204 = invoke class="VI" method="FP.Close"(reference=w418, error in=w419) -> (error out=w420:errorcluster)  [unwired: 1 in, 2 out]
              }
            }
          }
        }
        n205 = call <vilib>:"Add State(s) to Queue__jki_lib_state_machine.vi"("State(s) in (\"\")"=w398) -> ("States Out"=w397:string)  [unwired: 14 in]
      }
      frame "UI: Buttons" {
        # "Do not put any code in this frame.\n(It is a separator no-op. You can make a copy of this frame to create a new UI frame)"
        n206 = call <vilib>:"Add State(s) to Queue__jki_lib_state_machine.vi"("State(s) in (\"\")"=w424) -> ("States Out"=w423:string)  [unwired: 14 in]
      }
      frame "UI: Link Scroll Bars" {
        # "DON't"
        # "Do not put any code in this frame.\n(It is a separator no-op. You can make a copy of this frame to create a new UI frame)"
        n207 = control-ref of="AI"() -> (w435:refnum<vi>)
        n208 = control-ref of="Electrode"() -> (w434:refnum<vi>)
        n209 = control-ref of="Label"() -> (w433:refnum<vi>)
        n210 = control-ref of="Electrode Config"() -> (w432:refnum<vi>)
        n211 = control-ref of="KH #"() -> (w431:refnum<vi>)
        n212 = control-ref of="KH Configuration"() -> (w430:refnum<vi>)
        n213 = control-ref of="KH Gain"() -> (w429:refnum<vi>)
        n214 = control-ref of="KH Shunt Resistor"() -> (w428:refnum<vi>)
        n215 = control-ref of="Gain"() -> (w426:refnum<vi>)
        n216 = property class="Arr (strict)"(reference=w435) -> ("Index Values"=w425:u32[])  [unwired: 1 in, 2 out]
        n217 = property class="Arr (strict)"(reference=w434, "Index Values"=w425) -> ()  [unwired: 1 in, 2 out]
        n218 = property class="Arr (strict)"(reference=w433, "Index Values"=w425) -> ()  [unwired: 1 in, 2 out]
        n219 = property class="Arr (strict)"(reference=w432, "Index Values"=w425) -> ()  [unwired: 1 in, 2 out]
        n220 = property class="Arr (strict)"(reference=w431, "Index Values"=w425) -> ()  [unwired: 1 in, 2 out]
        n221 = property class="Arr (strict)"(reference=w430, "Index Values"=w425) -> ()  [unwired: 1 in, 2 out]
        n222 = property class="Arr (strict)"(reference=w429, "Index Values"=w425) -> ()  [unwired: 1 in, 2 out]
        n223 = property class="Arr (strict)"(reference=w428, "Index Values"=w425) -> ()  [unwired: 1 in, 2 out]
        n224 = property class="Arr (strict)"(reference=w426, "Index Values"=w425) -> ()  [unwired: 1 in, 2 out]
        n225 = property on="Scroll Bar" class="Arr (strict)"() -> ("Index Values"=w427:u32[])  [unwired: 2 in, 2 out]
        n226 = property on="Labels 2" class="Arr (strict)"("Index Values"=w427) -> ()  [unwired: 2 in, 2 out]
        n227 = property on="unused" class="Arr (strict)"("Index Values"=w427) -> ()  [unwired: 2 in, 2 out]
        n228 = property on="Electrodes 2" class="Arr (strict)"("Index Values"=w427) -> ()  [unwired: 2 in, 2 out]
        n229 = call <vilib>:"Add State(s) to Queue__jki_lib_state_machine.vi"("State(s) in (\"\")"=w439) -> ("States Out"=w438:string)  [unwired: 14 in]
      }
      frame "UI: SR Disable" {
        # "DONE"
        # "Do not put any code in this frame.\n(It is a separator no-op. You can make a copy of this frame to create a new UI frame)"
        n230 = local read "KH Addresses"() -> (w449:refnum<visa-resource-name>[])
        n231 = control-ref of="Shunt Resistor"() -> (w445:refnum<vi>)
        n232 = Index Array(array=w449) -> (element=w448:refnum<visa-resource-name>)  [unwired: 1 in]
        n233 = call <userlib>:"Shunt - Check 500 or 10M.vi"("error in (no error)"=w447, "VISA Refnum in"=w448) -> ("error out"=w446:errorcluster, "SR"=w442:enum16{"500", "10M"})  [unwired: 7 in, 1 out]
        n234 = call <vilib>:"Clear Errors.vi"("error in (no error)"=w446) -> ("error out"=w444:errorcluster)  [unwired: 5 in, 1 out]
        n235 = call <userlib>:"Shunt - 500 or 10M Control Disable.vi"("error in"=w444, "SR"=w442, "reference"=w445) -> ("error out"=w441:errorcluster)  [unwired: 8 in]
        n236 = control-ref of="Defualt Shunt Resistor"() -> (w443:refnum<vi>)
        n237 = call <userlib>:"Shunt - 500 or 10M Control Disable.vi"("error in"=w441, "SR"=w442, "reference"=w443) -> ("error out"=w440:errorcluster)  [unwired: 8 in]
        n238 = call <vilib>:"Add State(s) to Queue__jki_lib_state_machine.vi"("State(s) in (\"\")"=w452) -> ("States Out"=w451:string)  [unwired: 14 in]
      }
      frame "---------- Macro ----------" {
        # "Do not put any code in this frame.\n(It is a separator no-op. You can make a copy of this frame to create a new Macro frame)"
        n239 = call <vilib>:"Add State(s) to Queue__jki_lib_state_machine.vi"("State(s) in (\"\")"=w456) -> ("States Out"=w455:string)  [unwired: 14 in]
      }
      frame "Macro: Initialize" {
        # "Initialization Macro\n(This is called once, when the VI starts)"
        n240 = call <vilib>:"Add State(s) to Queue__jki_lib_state_machine.vi"("State(s) in Front (\"\")"="Data: Initialize\nInitialize Core Data\nData: Initialize Top Level\nData: Load Configuration\nUI: Update Controls\nUI: Initialize\nUI: Front Panel State >> Open\nUI: SR Disable\nExperiment VI: Populate VI Ring\n//Asana: Initialize Authentication Info\n//Macro: Asana\nPGSQL: Start Logger", "State(s) in (\"\")"=w461) -> ("States Out"=w460:string)  [unwired: 13 in]
      }
      frame "Macro: Exit" {
        # "Exit Macro\n(This is called once, when the VI exits)"
        n241 = Unbundle By Name(w469) -> ("Core.Close Panel on Exit?"=w468:bool)
        n242 = property on="OK" class="Bool (strict)"("Value"=FALSE ("Blinking")) -> ()  [unwired: 2 in, 2 out]
        n243 = Select(t="UI: Front Panel State >> Close", s=w468, f="") -> (s? t:f=w465:string)
        n244 = call <vilib>:"Add State(s) to Queue__jki_lib_state_machine.vi"("State(s) in (\"\")"=w465, "State(s) at Back (\"\")"="Data: Save Controls\nData: Cleanup\nExit") -> ("States Out"=w463:string)  [unwired: 13 in]
        n245 = call <vilib>:"Add State(s) to Queue__jki_lib_state_machine.vi"("State(s) in Front (\"\")"=w463, "State(s) in (\"\")"=w472) -> ("States Out"=w471:string)  [unwired: 13 in]
      }
      frame "Macro: Output" {
        # "#todo"
        n246 = case shown="True" "I'm Finished Taking Data!" {
          tunnel: [w487 _] -> w476
          frame False {
            n247 = local read "KH Addresses"() -> (w483:refnum<visa-resource-name>[])
            n248 = Empty Array?(array=w483) -> (empty?=w482:bool)
            n249 = Select(t="", s=w482, f="UI: SR Disable\nKH: set KH 0\nKH: set KH 1\nKH: set KH 2" ("State(s) in Front (\"\")")) -> (s? t:f=w484:string)
            n250 = call <vilib>:"Add State(s) to Queue__jki_lib_state_machine.vi"("State(s) in Front (\"\")"="Macro: Initialize Metadata" ("State(s) in Front (\"\")"), "State(s) in (\"\")"=w484, "State(s) at Back (\"\")"="Macro: Write Metadata" ("State(s) in Front (\"\")")) -> ("States Out"=w487:string)  [unwired: 12 in]
          }
          frame True {
          }
        }
        n251 = call <vilib>:"Add State(s) to Queue__jki_lib_state_machine.vi"("State(s) in Front (\"\")"=w476, "State(s) in (\"\")"=w479, "State(s) at Back (\"\")"="PGSQL: Write" ("State(s) in Front (\"\")")) -> ("States Out"=w478:string)  [unwired: 12 in]
      }
      frame "Macro: Initialize Metadata" {
        # "#todo"
        # "Do not put any code in this frame.\n(It is a separator no-op. You can make a copy of this frame to create a new Macro frame)"
        n252 = call <vilib>:"Add State(s) to Queue__jki_lib_state_machine.vi"("State(s) in Front (\"\")"="Metadata: Update Experiment Description\nMetadata: Update Wiring Configuration\nMetadata: Update KH\nMetadata: Build Path\nMetadata: Update Control Experiment Wire\nInstruments: Load Classes\nInstruments: Initialize KH\nInstruments: Initialize Lockin\nInstruments: Initialize Instruments" ("State(s) in Front (\"\")"), "State(s) in (\"\")"=w492) -> ("States Out"=w491:string)  [unwired: 13 in]
      }
      frame "Macro: Write Metadata" {
        # "#todo"
        # "Do not put any code in this frame.\n(It is a separator no-op. You can make a copy of this frame to create a new Macro frame)"
        n253 = call <vilib>:"Add State(s) to Queue__jki_lib_state_machine.vi"("State(s) in Front (\"\")"="Metadata: Update Comments\nMetadata: Update FGV\nMetadata: Write JSON\n//Macro: Asana" ("State(s) in Front (\"\")"), "State(s) in (\"\")"=w497) -> ("States Out"=w496:string)  [unwired: 13 in]
      }
      frame "Macro: Asana" {
        # "DON't"
        # "Do not put any code in this frame.\n(It is a separator no-op. You can make a copy of this frame to create a new Macro frame)"
        n254 = call <vilib>:"Add State(s) to Queue__jki_lib_state_machine.vi"("State(s) in Front (\"\")"="Asana: Authenticate\nAsana: Get Teams and Projects" ("State(s) in Front (\"\")"), "State(s) in (\"\")"=w502) -> ("States Out"=w501:string)  [unwired: 13 in]
      }
      frame "---------- Metadata ----------" {
        n255 = call <vilib>:"Add State(s) to Queue__jki_lib_state_machine.vi"("State(s) in (\"\")"=w506) -> ("States Out"=w505:string)  [unwired: 14 in]
      }
      frame "Metadata: Update Experiment Description" {
        # "DONE"
        n256 = Concatenate Strings("Sample (SAXXXX)", "." ("string"), "Device (YYYYMMDD)") -> (w510:string)
        n257 = Bundle By Name(cluster=w514, "Experiment.Device"=w510, "Experiment.User"="Username", "Experiment.Device Description"="Description", "Experiment.Instrument"="Instrument") -> (w515:T27)
        n258 = call <vilib>:"Add State(s) to Queue__jki_lib_state_machine.vi"("State(s) in (\"\")"=w518) -> ("States Out"=w517:string)  [unwired: 14 in]
      }
      frame "Metadata: Update Wiring Configuration" {
        # "DONE"
        n259 = local read "Lockin"() -> (w527:T7)
        n260 = local read "non KH"() -> (w521:T10)
        n261 = local read "Lockin"() -> (w525:T7)
        n262 = Unbundle By Name(w521) -> ("Electrodes 2"=w520:string[], "Labels 2"=w519:u16[])
        n263 = Unbundle By Name(w525) -> ("Electrode Config"=w524:T6[])
        n264 = Unbundle By Name(w527) -> ("AI"=w522:u32[], "Electrode"=w523:string[], "Label"=w526:u16[])
        n265 = for {
          tunnel: w519 -> [w536] mode=indexing
          tunnel: [w535] -> w528 mode=indexing
          n266 = property on="Ring" class="Ring (strict)"() -> ("Strings []"=w537:string[])  [unwired: 2 in, 2 out]
          n267 = Index Array(array=w537, index=w536) -> (element=w535:string)
        }
        n268 = for {
          tunnel: w526 -> [w539] mode=indexing
          tunnel: [w538] -> w529 mode=indexing
          n269 = property on="Ring" class="Ring (strict)"() -> ("Strings []"=w540:string[])  [unwired: 2 in, 2 out]
          n270 = Index Array(array=w540, index=w539) -> (element=w538:string)
        }
        n271 = Bundle By Name(cluster=w530, "Lockin Ch"=w522, "Electrodes"=w523, "Labels"=w529, "Electrodes"=w520, "Labels"=w528, "Lockin.Electrode Config"=w524) -> (w531:T27)
        n272 = call <vilib>:"Add State(s) to Queue__jki_lib_state_machine.vi"("State(s) in (\"\")"=w534) -> ("States Out"=w533:string)  [unwired: 14 in]
      }
      frame "Metadata: Update KH" {
        # "#todo\nin SMO?"
        # "I think this is obsolete with new control\ntype"
        n273 = local read "KH"() -> (w555:T5)
        n274 = local read "KH All Buttons"() -> (w556:T8)
        n275 = Unbundle By Name(w555) -> ("KH #"=w547:u16[], "KH Gain"=w551:T3[], "KH Configuration"=w550:T2[], "KH Shunt Resistor"=w546:T4[])
        n276 = call "Initialize KH Array.vi"("KH #"=w547, "Control in"=w551) -> ("Control out"=w554:variant)  [unwired: 9 in]
        n277 = Variant To Data(error in=w542, type=w551, Variant=w554) -> (data=w553:T3[], error out=w541:errorcluster)
        n278 = call "Initialize KH Array.vi"("KH #"=w547, "Control in"=w550) -> ("Control out"=w552:variant)  [unwired: 9 in]
        n279 = Variant To Data(error in=w541, type=w550, Variant=w552) -> (data=w549:T2[], error out=w543:errorcluster)
        n280 = call "Initialize KH Array.vi"("KH #"=w547, "Control in"=w546) -> ("Control out"=w548:variant)  [unwired: 9 in]
        n281 = Variant To Data(error in=w543, type=w546, Variant=w548) -> (data=w545:T4[], error out=w544:errorcluster)
        n282 = Bundle By Name(cluster=w557, "KH.KH #"=w547, "KH.KH Gain"=w553, "KH.KH Configuration"=w549, "KH.KH Shunt Resistor"=w545, "KH All Buttons"=w556) -> (w558:T27)
        n283 = call <vilib>:"Add State(s) to Queue__jki_lib_state_machine.vi"("State(s) in (\"\")"=w560) -> ("States Out"=w559:string)  [unwired: 14 in]
      }
      frame "Metadata: Build Path" {
        # "DONE"
        n284 = Unbundle By Name(w572) -> ("Experiment.Instrument"=w569:T9, "Experiment.Device"=w567:string)  [unwired: 1 out]
        n285 = Format Into String(w569) -> (resulting string=w568:string)  [unwired: 3 in, 1 out]
        n286 = Build Path(base path="Default Path", name or relative path=w568) -> (appended path=w570:path)
        n287 = Build Path(base path=w570, name or relative path=w567) -> (appended path=w566:path)
        n288 = call <userlib>:"MGI Create Directory Chain.vi"("Error In"=w565, "File Presence (Auto Detect)"=MGI_Create_Directory_Chain_Behavior_Enum."Path Does Not Contain a File", "Path"=w566) -> ("Error Out"=w564:errorcluster, "Duplicate Path"=w562:path)  [unwired: 7 in]
        "Device Folder" <- w562
        n289 = Bundle By Name(cluster=w572, "Experiment.Device Path"=w562) -> (w571:T27)
        n290 = call <vilib>:"Add State(s) to Queue__jki_lib_state_machine.vi"("State(s) in (\"\")"=w574) -> ("States Out"=w573:string)  [unwired: 14 in]
      }
      frame "Metadata: Update Control Experiment Wire" {
        # "DONE"
        # "IS Control Experiment Class wire"
        # "Not on Control Experiment Class wire"
        n291 = Unbundle By Name(w579) -> ("C.E."=w577:refnum<class "Control Experiment SM.lvclass">, "Experiment"=w581:T22, "Wiring"=w580:T23)
        n292 = Bundle By Name(cluster=w577, "Experiment"=w581, "Wiring"=w580) -> (w575:refnum<class "Control Experiment SM.lvclass">)
        n293 = Bundle By Name(cluster=w579, "C.E."=w575) -> (w578:T27)
        n294 = call <vilib>:"Add State(s) to Queue__jki_lib_state_machine.vi"("State(s) in (\"\")"=w583) -> ("States Out"=w582:string)  [unwired: 14 in]
      }
      frame "Metadata: Update Comments" {
        # "#todo\nin SMO"
        # "#todo"
        # "error 63 occurs when\nthe lockin isn't running\nI think we can clear here?"
        n295 = Unbundle By Name(w594) -> ("C.E."=w590:refnum<class "Control Experiment SM.lvclass">)
        n296 = call "Generate Comments.vi"("error in (no error)"=w585, "Control Experiment"=w590) -> ("error out"=w587:errorcluster, "Control Experiment out"=w589:refnum<class "Control Experiment SM.lvclass">)  [unwired: 6 in, 1 out]
        n297 = call <vilib>:"Clear Errors.vi"("error in (no error)"=w587, "specific error code to clear (0: all)"=63) -> ("error out"=w586:errorcluster)  [unwired: 4 in, 1 out]
        n298 = call "Read Comments.vi"("error in (no error)"=w586, "Control Experiment in"=w589) -> ("error out"=w584:errorcluster, "Comments"=→"Comments":string, "Control Experiment out"=w591:refnum<class "Control Experiment SM.lvclass">)  [unwired: 7 in]
        n299 = Bundle By Name(cluster=w594, "C.E."=w591) -> (w593:T27)
        n300 = call <vilib>:"Add State(s) to Queue__jki_lib_state_machine.vi"("State(s) in (\"\")"=w596) -> ("States Out"=w595:string)  [unwired: 14 in]
      }
      frame "Metadata: Update FGV" {
        # "DONE"
        n301 = Unbundle By Name(w601) -> ("C.E."=w598:refnum<class "Control Experiment SM.lvclass">)
        n302 = call "Control Experiment FGV.vi"("Function"=enum16{"read", "write"}."write", "error in (no error)"=w597, "Control Experiment.lvclass"=w598) -> ("error out"=w599:errorcluster)  [unwired: 7 in, 1 out]
        n303 = call <vilib>:"Add State(s) to Queue__jki_lib_state_machine.vi"("State(s) in (\"\")"=w603) -> ("States Out"=w602:string)  [unwired: 14 in]
      }
      frame "Metadata: Write JSON" {
        w610 = T31 {"Device"={"Device"="", "User"="", "Time"="", "Computer Name"=""}, "Wiring"={"Lockin Ch"=[], "KH Electrodes"=[], "KH Labels"=[], "Other Electrodes"=[], "Other Labels"=[]}}  # Control Experiment JSON
        # "#todo\nin SMO"
        # "#todo"
        n304 = Unbundle By Name(w620) -> ("C.E."=w611:refnum<class "Control Experiment SM.lvclass">, "Experiment.Device"=w625:string, "Experiment.User"=w624:string)
        n305 = call "Get Date Time ISO.vi"("error in (no error)"=w617) -> ("error out"=w606:errorcluster, "ISO 8601 date-time string"=w616:string)  [unwired: 8 in, 1 out]
        n306 = Unbundle By Name(w620) -> ("Lockin.AI"=w623:u32[], "Electrodes"=w622, "Labels"=w621, "Electrodes"=w619, "Labels"=w618)
        n307 = call "Get Local Computer Name.vi"("error in (no error)"=w606) -> ("error out"=w605:errorcluster, "Name"=w604:string)  [unwired: 8 in, 1 out]
        n308 = Bundle By Name(cluster=w610, "Device.Device"=w625, "Device.User"=w624, "Device.Time"=w616, "Device.Computer Name"=w604) -> (w609:T31)
        n309 = Bundle By Name(cluster=w609, "Wiring.Lockin Ch"=w623, "Wiring.KH Electrodes"=w622, "Wiring.KH Labels"=w621, "Wiring.Other Electrodes"=w619, "Wiring.Other Labels"=w618) -> (w608:T31)
        n310 = call <vilib>:"Flatten To JSON String.vi"("Enums As String (F)"=TRUE, "error in (no error)"=w605, "Variant"=w608) -> ("error out"=w613:errorcluster, "JSON String"=→"JSON String":string)  [unwired: 7 in]
        n311 = call "Write Experiment Folder.vi"("error in (no error)"=w613, "Experiment Folder"="device", "Control Experiment in"=w611) -> ("error out"=w612:errorcluster, "Control Experiment out"=w614:refnum<class "Control Experiment SM.lvclass">)  [unwired: 7 in]
        n312 = call "Save JSON File.vi"("error in (no error)"=w612, "Data"=w608, "Control Experiment in"=w614) -> ("error out"=w615:errorcluster)  [unwired: 6 in, 2 out]
        n313 = call <vilib>:"Add State(s) to Queue__jki_lib_state_machine.vi"("State(s) in (\"\")"=w629) -> ("States Out"=w628:string)  [unwired: 14 in]
      }
      frame "---------- KH ----------" {
        n314 = call <vilib>:"Add State(s) to Queue__jki_lib_state_machine.vi"("State(s) in (\"\")"=w633) -> ("States Out"=w632:string)  [unwired: 14 in]
      }
      frame "KH: set KH 0" {
        # "DONE"
        # "already done"
        # "initialize the Channel Settings array"
        # "remove duplicates"
        n315 = local read "KH Addresses"() -> (w646:refnum<visa-resource-name>[])
        n316 = call-poly <userlib>:"Remove Duplicates from 1D Array__ogtk.vi"("Input Array"=w646) -> ("Output Array"=w647:variant[])  [unwired: 1 out]
        n317 = Variant To Data(error in=w645, type=w646, Variant=w647) -> (data=w638:refnum<visa-resource-name>[], error out=w637:errorcluster)
        n318 = local write "KH Addresses"(w638) -> ()
        n319 = Initialize Array(T16 {"Channel"=enum."Channel 1", "Gain"=enum."10x", "Bandwidth Filter"=enum."ON", "Shunt Resistor"=enum."50 Ohms", "Coupling"=enum."DC", "Input Config"=enum."Differential"} ("Channel Settings"), 8 ("dimension size")) -> (w640:T16[])
        n320 = Bundle(w640) -> (w639:cluster{T16[]})  [unwired: 1 in]
        n321 = Array Size(array=w638) -> (size(s)=w643:i32)
        n322 = for {
          tunnel: w638 -> [_] mode=indexing
          tunnel: [w655] -> w634 mode=concatenating
          tunnel: w637 -> [w654]
          tunnel: [w653] -> w636
          i -> [w657]
          n323 = call "Number to Letter.vi"("Number"=w657) -> ("Letter"=w656:string)
          n324 = for {
            N: 8 -> [_]
            tunnel: w656 -> [w662]
            tunnel: [w661] -> w655 mode=indexing
            tunnel: w654 -> [w660]
            tunnel: [w659] -> w653
            i -> [w664]
            n325 = Increment(x=w664) -> (x+1=w658:i32)
            n326 = Format Into String(format string="%s %d", error in=w660, w662, w658) -> (resulting string=w661:string, error out=w659:errorcluster)  [unwired: 1 in]
          }
        }
        n327 = Initialize Array(w639, w643) -> (w644:cluster{T16[]}[])
        n328 = Bundle By Name(cluster=w649, "Channel Settings"=w644) -> (w648:T27)
        n329 = property on="Ring" class="Ring (strict)"(error in=w636, "Strings []"=w634) -> (error out=w635:errorcluster)  [unwired: 1 in, 1 out]
        n330 = call <vilib>:"Add State(s) to Queue__jki_lib_state_machine.vi"("State(s) in (\"\")"=w651) -> ("States Out"=w650:string)  [unwired: 14 in]
      }
      frame "KH: set KH 1" {
        # "DONE"
        n331 = Unbundle By Name(w676) -> ("Channel Settings"=w665:cluster{"Channel Setting":T24}[], "KH.KH #"=w678:u16[], "KH.KH Gain"=w681:T3[], "Lockin.Electrode Config"=w679:T6[], "KH.KH Shunt Resistor"=w680:T4[], "KH All Buttons"=w677:T8)
        n332 = local read "Bandwidth Filter"() -> (w666:bool)
        n333 = local read "DC Coupled"() -> (w667:bool)
        n334 = for {
          tunnel: w679 -> [w706] mode=indexing
          tunnel: w681 -> [w705] mode=indexing
          tunnel: w680 -> [w704] mode=indexing
          tunnel: w678 -> [w700] mode=indexing
          tunnel: [w709] -> w672 mode=indexing
          tunnel: w677 -> [w708]
          tunnel: [w707] -> w670 mode=indexing
          tunnel: [w703] -> w671 mode=indexing
          shift-right: [w696] -> w674
          shift-left: w665 -> [w697]
          tunnel: w667 -> [w692]
          tunnel: w666 -> [w687]
          n335 = property on="Ring" class="Ring (strict)"() -> ("Strings []"=w702:string[])  [unwired: 2 in, 2 out]
          n336 = case shown="\"All Differential\"" w708 {
            tunnel: w706 -> [w728 _ _]
            tunnel: [w733 Input_Configuration-Enum."Ground" ("Input Config") Input_Configuration-Enum."Differential" ("Input Config")] -> w703
            tunnel: w705 -> [w732 w751 w754]
            tunnel: [w731 w751 w754] -> w707
            tunnel: w704 -> [w730 _ _]
            tunnel: [w729 Shunt-Enum."Open" ("Shunt Resistor") w752] -> w709
            frame "No Selection", Default {
              n337 = case shown="\"Voltage (SE)\"" w728 {
                tunnel: [Input_Configuration-Enum."Ground" ("Input Config") Input_Configuration-Enum."Differential" ("Input Config") Input_Configuration-Enum."SE+ (-gnd)" ("Input Config") Input_Configuration-Enum."Differential" ("Input Config") Input_Configuration-Enum."Differential" ("Input Config")] -> w733
                tunnel: [Shunt-Enum."Open" ("Shunt Resistor") w737 Shunt-Enum."Open" ("Shunt Resistor") Shunt-Enum."Open" ("Shunt Resistor") Shunt-Enum."50k Ohms" ("Shunt Resistor")] -> w729
                tunnel: w732 -> [w734 w738 w741 w745 w747]
                tunnel: [w734 w738 w741 w745 w747] -> w731
                tunnel: w730 -> [_ w737 _ _ _]
                frame "Ground", Default {
                }
                frame "Current" {
                }
                frame "Voltage (SE)" {
                }
                frame "Voltage (Diff)" {
                }
                frame "Gate" {
                }
              }
            }
            frame "All Ground" {
            }
            frame "All Differential" {
              n338 = local read "Defualt Shunt Resistor"() -> (w752:T4)
            }
          }
          n339 = To Long Integer(number=w700) -> (32bit integer=w701:i32)
          n340 = Index Array(array=w702, index=w701) -> (element=w699:string)
          n341 = Select(t=Coupling-Enum."DC" ("Coupling"), s=w692, f=Coupling-Enum."AC" ("Coupling")) -> (s? t:f=w689:T19)
          n342 = Scan From String(format string="%s %d", input string=w699) -> (error out=w693:errorcluster, output 1=w695:string, output 2=w694:i32)  [unwired: 4 in, 2 out]
          n343 = Select(t=Filter-Enum."ON" ("Bandwidth Filter"), s=w687, f=Filter-Enum."OFF" ("Bandwidth Filter")) -> (s? t:f=w685:T18)
          n344 = case shown="No Error" w693 {
            tunnel: w709 -> [w726 _]
            tunnel: w707 -> [w725 _]
            tunnel: w703 -> [w724 _]
            tunnel: w697 -> [w716 w727]
            tunnel: [w715 w727] -> w696
            tunnel: w695 -> [w714 _]
            tunnel: w694 -> [w713 _]
            tunnel: w689 -> [w711 _]
            tunnel: w685 -> [w710 _]
            frame No Error {
              n345 = Decrement(x=w713) -> (x-1=w712:i32)
              n346 = call "Letter to Number.vi"("Letter"=w714) -> ("Number"=w717:i32)
              n347 = Index Array(array=w716, index=w717) -> (element=w722:cluster{"Channel Setting":T24})
              n348 = Unbundle(w722) -> ("Channel Setting"=w721:T24)
              n349 = Index Array(array=w721, index=w712) -> (element=w720:T16)
              n350 = Bundle By Name(cluster=w720, "Channel"=w712, "Gain"=w725, "Input Config"=w724, "Shunt Resistor"=w726, "Coupling"=w711, "Bandwidth Filter"=w710) -> (w719:T16)
              n351 = Replace Array Subset(array=w721, new element=w719, index=w712) -> (w723:T24)
              n352 = Bundle("Channel Setting"=w723) -> (w718:cluster{"Channel Setting":T24})  [unwired: 1 in]
              n353 = Replace Array Subset(array=w716, new element=w718, index=w717) -> (w715:cluster{"Channel Setting":T24}[])
            }
            frame Error {
            }
          }
        }
        n354 = local write "KH All Buttons"(T8."No Selection" ("KH All Buttons")) -> ()
        n355 = Bundle By Name(cluster=w676, "Channel Settings"=w674, "KH.KH Gain"=w670, "KH.KH Configuration"=w671, "KH.KH Shunt Resistor"=w672) -> (w682:T27)
        n356 = local read "KH"() -> (w673:T5)
        n357 = Bundle By Name(cluster=w673, "KH Gain"=w670, "KH Configuration"=w671, "KH Shunt Resistor"=w672) -> (w669:T5)
        n358 = local write "KH"(w669) -> ()
        n359 = call <vilib>:"Add State(s) to Queue__jki_lib_state_machine.vi"("State(s) in (\"\")"=w684) -> ("States Out"=w683:string)  [unwired: 14 in]
      }
      frame "KH: set KH 2" {
        # "DONE"
        n360 = Unbundle By Name(w764) -> ("Channel Settings"=w767:cluster{"Channel Setting":T24}[])
        n361 = Unbundle By Name(w764) -> ("C.E."=w762:refnum<class "Control Experiment SM.lvclass">)
        n362 = Unbundle By Name(w762) -> ("KH7008"=w761:refnum<class "Instrument.KH7008.lvclass">[])
        n363 = for {
          tunnel: w760 -> [w782]
          tunnel: [w774] -> w755
          tunnel: w767 -> [w781] mode=indexing
          tunnel: w761 -> [w780] mode=indexing
          tunnel: [w773] -> w765 mode=concatenating
          tunnel: [w772] -> w759 mode=indexing
          n364 = Unbundle(w781) -> ("Channel Setting"=w777:T24)
          n365 = call <userlib>:"Write Channel Setting.vi"("error in (no error)"=w782, "Channel Setting"=w777, "KH7008 in"=w780) -> ("error out"=w778:errorcluster, "KH7008 out"=w779:refnum<class "Instrument.KH7008.lvclass">)  [unwired: 7 in]
          n366 = call <userlib>:"KH Control.vi"("error in"=w778, "KH7008.lvclass"=w779) -> ("error out"=w776:errorcluster, "KH7008.lvclass out"=w775:refnum<class "Instrument.KH7008.lvclass">)  [unwired: 8 in]
          n367 = call <userlib>:"Read Gain.vi"("error in (no error)"=w776, "KH7008 in"=w775) -> ("error out"=w774:errorcluster, "Gain"=w773:dbl[], "KH7008 out"=w772:refnum<class "Instrument.KH7008.lvclass">)  [unwired: 7 in]
        }
        n368 = local read "Gain"() -> (w766:dbl[])
        n369 = Bundle By Name(cluster=w762, "KH7008"=w759) -> (w763:refnum<class "Control Experiment SM.lvclass">)
        n370 = call "Multiply Gains.vi"("Other Gain"=w766, "Gain"=w765) -> ("Gain x Other Gain"=w757:dbl[])
        n371 = Unbundle By Name(w763) -> ("Lockin"=w758:refnum<class "Instrument.Lockin.lvclass">)
        n372 = call <userlib>:"setInputGain.vi"("error in (no error)"=w755, "InputGain"=w757, "Instrument.Lockin in"=w758) -> ("error out"=w756:errorcluster)  [unwired: 7 in, 1 out]
        n373 = Bundle By Name(cluster=w764, "C.E."=w763) -> (w769:T27)
        n374 = call <vilib>:"Clear Errors.vi"("error in (no error)"=w756) -> ("error out"=w768:errorcluster)  [unwired: 5 in, 1 out]
        n375 = call <vilib>:"Add State(s) to Queue__jki_lib_state_machine.vi"("State(s) in (\"\")"=w771) -> ("States Out"=w770:string)  [unwired: 14 in]
      }
      frame "---------- Instruments ----------" {
        n376 = call <vilib>:"Add State(s) to Queue__jki_lib_state_machine.vi"("State(s) in (\"\")"=w786) -> ("States Out"=w785:string)  [unwired: 14 in]
      }
      frame "Instruments: Load Classes" {
        # "DONE"
        n377 = Unbundle By Name(w792) -> ("C.E."=w790:refnum<class "Control Experiment SM.lvclass">)
        n378 = call "Load Instrument Classes.vi"("error in (no error)"=w787, "Control Experiment.lvclass"=w790) -> ("error out"=w788:errorcluster, "Control Experiment out"=w789:refnum<class "Control Experiment SM.lvclass">)  [unwired: 8 in]
        n379 = Bundle By Name(cluster=w792, "C.E."=w789) -> (w791:T27)
        n380 = call <vilib>:"Add State(s) to Queue__jki_lib_state_machine.vi"("State(s) in (\"\")"=w794) -> ("States Out"=w793:string)  [unwired: 14 in]
      }
      frame "Instruments: Initialize KH" {
        # "DONE"
        n381 = Unbundle By Name(w798) -> ("C.E."=w799:refnum<class "Control Experiment SM.lvclass">)
        n382 = Unbundle By Name(w799) -> ("KH7008"=w801:refnum<class "Instrument.KH7008.lvclass">[])
        n383 = for {
          tunnel: w801 -> [w807]
          tunnel: [w811] -> w795 mode=indexing
          tunnel: w803 -> [w810]
          tunnel: [w809] -> w802
          tunnel: "KH Addresses" -> [w808] mode=indexing
          n384 = Index Array(array=w807) -> (element=w806:refnum<class "Instrument.KH7008.lvclass">)  [unwired: 1 in]
          n385 = call-dynamic "Open.vi"("error in (no error)"=w810, "Address"=w808, "Instrument.KH7008 in"=w806) -> ("error out"=w809:errorcluster, "Instrument.KH7008 out"=w811:refnum<class "Instrument.KH7008.lvclass">)  [unwired: 7 in]
        }
        n386 = Bundle By Name(cluster=w799, "KH7008"=w795) -> (w796:refnum<class "Control Experiment SM.lvclass">)
        n387 = Bundle By Name(cluster=w798, "C.E."=w796) -> (w797:T27)
        n388 = call <vilib>:"Add State(s) to Queue__jki_lib_state_machine.vi"("State(s) in (\"\")"=w805) -> ("States Out"=w804:string)  [unwired: 14 in]
      }
      frame "Instruments: Initialize Lockin" {
        # "DONE"
        n389 = Unbundle By Name(w818) -> ("C.E."=w814:refnum<class "Control Experiment SM.lvclass">)
        n390 = Unbundle By Name(w814) -> ("Lockin"=w815:refnum<class "Instrument.Lockin.lvclass">)
        n391 = call-dynamic "Open.vi"("error in (no error)"=w819, "Address"="Lockin Address", "Instrument.Lockin in"=w815) -> ("error out"=w816:errorcluster, "Instrument.Lockin out"=w813:refnum<class "Instrument.Lockin.lvclass">)  [unwired: 7 in]
        n392 = Bundle By Name(cluster=w814, "Lockin"=w813) -> (w812:refnum<class "Control Experiment SM.lvclass">)
        n393 = Bundle By Name(cluster=w818, "C.E."=w812) -> (w817:T27)
        n394 = call <vilib>:"Add State(s) to Queue__jki_lib_state_machine.vi"("State(s) in (\"\")"=w822) -> ("States Out"=w821:string)  [unwired: 14 in]
      }
      frame "Instruments: Initialize Instruments" {
        # "DONE"
        n395 = Unbundle By Name(w827) -> ("C.E."=w826:refnum<class "Control Experiment SM.lvclass">)
        n396 = Unbundle By Name(w826) -> ("C Bridge"=w834:refnum<class "Instrument.CBridge.lvclass">, "Strain Cell"=w832:refnum<class "Instrument.Strain.lvclass">)
        n397 = call-dynamic "Open.vi"("error in (no error)"=w829, "Address"="Capacitance Bridge Address", "Instrument in"=w834) -> ("error out"=w833:errorcluster, "Instrument out"=w825:refnum<class "Instrument.CBridge.lvclass">)  [unwired: 7 in]
        n398 = call-dynamic "Open.vi"("error in (no error)"=w833, "Address"="Strain Cell Address", "Instrument in"=w832) -> ("error out"=w828:errorcluster, "Instrument out"=w824:refnum<class "Instrument.Strain.lvclass">)  [unwired: 7 in]
        n399 = Bundle By Name(cluster=w826, "C Bridge"=w825, "Strain Cell"=w824) -> (w823:refnum<class "Control Experiment SM.lvclass">)
        n400 = Bundle By Name(cluster=w827, "C.E."=w823) -> (w835:T27)
        n401 = call <vilib>:"Add State(s) to Queue__jki_lib_state_machine.vi"("State(s) in (\"\")"=w837) -> ("States Out"=w836:string)  [unwired: 14 in]
      }
      frame "---------- Asana ----------" {
        n402 = call <vilib>:"Add State(s) to Queue__jki_lib_state_machine.vi"("State(s) in (\"\")"=w841) -> ("States Out"=w840:string)  [unwired: 14 in]
      }
      frame "Asana: Initialize Authentication Info" {
        # "DON't"
        n403 = Bundle By Name(cluster=w843, "Asana.Authentication Info.Client ID"="1150712142949183" ("Client ID"), "Asana.Authentication Info.Client Secret"="530770942aed47201cd52aeb331bdd57" ("Client Secret"), "Asana.Authentication Info.Redirect URI"="https://www.google.com/" ("Redirect URI")) -> (w842:T27)
        n404 = call <vilib>:"Add State(s) to Queue__jki_lib_state_machine.vi"("State(s) in (\"\")"=w849) -> ("States Out"=w848:string)  [unwired: 14 in]
      }
      frame "Asana: Authenticate" {
        # "DON't"
        n405 = Unbundle By Name(w851) -> ("Asana.Time Stamp"=w865:timestamp, "Asana.Refresh Token"=w852:string, "Asana.Authentication Info"=w855:T32)
        n406 = Get Date/Time In Seconds() -> (seconds since 1Jan1904=w864:timestamp)
        n407 = Subtract(x=w865, y=w864) -> (x-y=w863:dbl)
        n408 = Less?(x=w863, y=3600.0) -> (x < y?=w856:bool)
        n409 = Select(t=w852, s=w856, f="" ("t")) -> (s? t:f=w854:string)
        n410 = call <userlib>:"Asana Authentication.vi"("error in (no error)"=w850, "Authentication Info"=w855, "Refresh Token In"=w854) -> ("error out"=w859:errorcluster, "Authentication Header"=w858:T26[], "Refresh Token Out"=w857:string)  [unwired: 5 in, 1 out]
        n411 = case shown="Error" w859 {
          selector: w859 -> [w869 _]
          tunnel: w858 -> [w870 _]
          tunnel: w857 -> [w868 _]
          tunnel: w851 -> [w873 w875]
          tunnel: [w871 w875] -> w861
          tunnel: [w869 errorcluster {"status"=FALSE, "code"=0, "source"=""} ("error in (no error)")] -> w860
          frame No Error {
            n412 = Get Date/Time In Seconds() -> (seconds since 1Jan1904=w872:timestamp)
            n413 = Bundle By Name(cluster=w873, "Asana.Refresh Token"=w868, "Asana.Authentication Header"=w870, "Asana.Time Stamp"=w872) -> (w871:T27)
            "Refresh Token Out" <- w868
          }
          frame Error {
          }
        }
        n414 = call <vilib>:"Add State(s) to Queue__jki_lib_state_machine.vi"("State(s) in (\"\")"=w867) -> ("States Out"=w866:string)  [unwired: 14 in]
      }
      frame "Asana: Get Teams and Projects" {
        # "DON't"
        # "task"
        # "project"
        # "team"
        n415 = Unbundle By Name(w883) -> ("Asana.Authentication Header"=w879:T26[])
        n416 = Unbundle By Name(w883) -> ("Experiment.Device"=w876:string)
        n417 = call <userlib>:"Get Teams.vi"("Authorization"=w879, "error in (no error)"=w896) -> ("error out"=w895:errorcluster, "Teams Out"=w885:T33)  [unwired: 8 in]
        n418 = Format Into String(error in=w895, T20."Samples" ("Team")) -> (resulting string=w894:string, error out=w893:errorcluster)  [unwired: 2 in]
        n419 = call "Asana Dictionary Get Value.vi"("error in (no error)"=w893, "Key"=w894, "Data"=w885) -> ("error out"=w890:errorcluster, "Value"=w892:string)  [unwired: 7 in]
        n420 = call <userlib>:"Get Projects.vi"("Authorization"=w879, "error in (no error)"=w890, "Team GID"=w892) -> ("error out"=w889:errorcluster, "Projects Out"=w887:T33)  [unwired: 7 in]
        n421 = call "Asana Dictionary Get Value.vi"("error in (no error)"=w889, "Key"="Devices" ("element"), "Data"=w887) -> ("error out"=w888:errorcluster, "Value"=w877:string)  [unwired: 7 in]
        n422 = call <userlib>:"Get Tasks.vi"("Authorization"=w879, "error in (no error)"=w888, "Project GID"=w877) -> ("error out"=w884:errorcluster, "data"=w886:T34)  [unwired: 7 in]
        n423 = call "Asana Dictionary Tasks Get Value.vi"("error in (no error)"=w884, "Key"=w876, "data"=w886) -> ("error out"=w881:errorcluster, "Value"=w882:string)  [unwired: 7 in]
        n424 = case shown="\"\"" w882 {
          tunnel: w881 -> [w899 w904]
          tunnel: [w899 w903] -> w880
          tunnel: w879 -> [_ w902]
          tunnel: w877 -> [_ w901]
          tunnel: w876 -> [_ w900]
          frame Default {
          }
          frame "" {
            # "empty means\ntask doesn't\nexist"
            n425 = case shown="Default" w900 {
              selector: w900 -> [_ w906]
              tunnel: w904 -> [w905 w910]
              tunnel: [w905 w909] -> w903
              tunnel: w902 -> [_ w908]
              tunnel: w901 -> [_ w907]
              frame "" {
              }
              frame Default {
                n426 = call <userlib>:"Create Task.vi"("Authorization"=w908, "error in (no error)"=w910, "Name"=w906, "Project GID"=w907) -> ("error out"=w909:errorcluster)  [unwired: 6 in, 1 out]
              }
            }
          }
        }
        n427 = call <vilib>:"Add State(s) to Queue__jki_lib_state_machine.vi"("State(s) in (\"\")"=w898) -> ("States Out"=w897:string)  [unwired: 14 in]
      }
      frame "---------- Experiment VI ----------" {
        n428 = call <vilib>:"Add State(s) to Queue__jki_lib_state_machine.vi"("State(s) in (\"\")"=w914) -> ("States Out"=w913:string)  [unwired: 14 in]
      }
      frame "Experiment VI: Populate VI Ring" {
        # "DONE"
        n429 = call <userlib>:"Current VIs Parent Directory__ogtk.vi"() -> ("Parent Directory (+ Relative)"=w931:path)  [unwired: 5 in]
        n430 = call <userlib>:"String to 1D Array__ogtk.vi"("delimiter (Tab)"="\n", "string"="----Sweep Control----\nSweep Control.vi\nContinuous B Sweep.vi") -> ("Array of Strings"=w917:string[])  [unwired: 9 in]
        n431 = call <userlib>:"String to 1D Array__ogtk.vi"("delimiter (Tab)"="\n", "string"="----Transport----\nIV.vi\nIV_Sweep.vi\nLockin_time.vi\nLockin_Vsg.vi\nLockin_sweep.vi\nLockin_AIWFM_time.vi\nTHz_TimeDelay.vi\nSweep_AIWFM_time.vi") -> ("Array of Strings"=w916:string[])  [unwired: 9 in]
        n432 = Strip Path(path=w931) -> (stripped path=w928:path)  [unwired: 1 out]
        n433 = Build Path(base path=w928, name or relative path="SweepControl") -> (appended path=w927:path)
        n434 = Build Path(base path=w928, name or relative path="Transport") -> (appended path=w923:path)
        n435 = for {
          tunnel: w927 -> [w941]
          tunnel: w917 -> [w940] mode=indexing
          tunnel: [w939] -> w920 mode=indexing
          n436 = Build Path(base path=w941, name or relative path=w940) -> (appended path=w939:path)
        }
        n437 = for {
          tunnel: w923 -> [w938]
          tunnel: w916 -> [w937] mode=indexing
          tunnel: [w936] -> w919 mode=indexing
          n438 = Build Path(base path=w938, name or relative path=w937) -> (appended path=w936:path)
        }
        n439 = Build Array (concatenate)(w920, w919) -> (w918:path[])
        n440 = Build Array (concatenate)(w917, w916) -> (w915:string[])
        n441 = Bundle By Name(cluster=w922, "VI paths"=w918) -> (w921:T27)
        n442 = property on="Ring" class="Ring (strict)"("Strings []"=w915) -> ()  [unwired: 2 in, 2 out]
        n443 = call <vilib>:"Add State(s) to Queue__jki_lib_state_machine.vi"("State(s) in (\"\")"=w935) -> ("States Out"=w934:string)  [unwired: 14 in]
      }
      frame "Experiment VI: Open VI" {
        # "DONE"
        n444 = Unbundle By Name(w947) -> ("VI paths"=w946:path[])
        n445 = Index Array(array=w946, index="Ring") -> (element=w944:path)
        n446 = call "Open Experiment VI.vi"("error in (no error)"=w943, "Path"=w944) -> ("error out"=w942:errorcluster)  [unwired: 9 in]
        n447 = call <vilib>:"Add State(s) to Queue__jki_lib_state_machine.vi"("State(s) in (\"\")"=w949) -> ("States Out"=w948:string)  [unwired: 14 in]
      }
      frame "Experiment VI: Open Lockin" {
        # "DONE"
        n448 = call "Open Lockin.vi"("error in (no error)"=w951) -> ("error out"=w950:errorcluster)  [unwired: 10 in]
        n449 = call <vilib>:"Add State(s) to Queue__jki_lib_state_machine.vi"("State(s) in (\"\")"=w954) -> ("States Out"=w953:string)  [unwired: 14 in]
      }
      frame "---------- PGSQL ----------" {
        n450 = call <vilib>:"Add State(s) to Queue__jki_lib_state_machine.vi"("State(s) in (\"\")"=w958) -> ("States Out"=w957:string)  [unwired: 14 in]
      }
      frame "PGSQL: Start Logger" {
        # "DON't"
        n451 = Unbundle By Name(w960) -> ("Logger"=w965:refnum<class "Logger.PGSQL.lvclass">)
        n452 = call <vilib>:"Create.vi"("error in (no error)"=w962, "SMO"=w965) -> ("error out"=w964:errorcluster, "SMO out"=w966:refnum<class "Logger.PGSQL.lvclass">)  [unwired: 7 in, 1 out]
        n453 = call <vilib>:"Start.vi"("error in (no error)"=w964, "SMO"=w966) -> ("error out"=w961:errorcluster, "SMO out"=w963:refnum<class "Logger.PGSQL.lvclass">)  [unwired: 8 in]
        n454 = Bundle By Name(cluster=w960, "Logger"=w963) -> (w959:T27)
        n455 = call <vilib>:"Add State(s) to Queue__jki_lib_state_machine.vi"("State(s) in (\"\")"=w968) -> ("States Out"=w967:string)  [unwired: 14 in]
      }
      frame "PGSQL: Write" {
        w980 = "" ("f")
        # "DONE"
        n456 = Unbundle By Name(w984) -> ("Logger"=w978:refnum<class "Logger.PGSQL.lvclass">, "Experiment.Instrument"=w969:T9, "Experiment.Device"=w983:string, "Experiment.User"=w982:string)
        n457 = local read "I'm Finished Taking Data!"() -> (w981:bool)
        n458 = Not(x=w981) -> (.not. x?=w979:bool)
        n459 = call "Device and User PGSQL Paths.vi"("instrument"=w969) -> ("User Path"=w971:string, "Device Path"=w977:string)  [unwired: 5 in]
        n460 = Select(t=w983, s=w979, f=w980) -> (s? t:f=w976:string)
        n461 = Select(t=w982, s=w979, f=w980) -> (s? t:f=w970:string)
        n462 = call <userlib>:"Logger.PGSQL.WriteVariable.vi"("error in (no error)"=w974, "Data"=w976, "Address"=w977, "Logger"=w978) -> ("error out"=w973:errorcluster, "Logger out"=w975:refnum<class "Logger.PGSQL.lvclass">)  [unwired: 6 in]
        n463 = call <userlib>:"Logger.PGSQL.WriteVariable.vi"("error in (no error)"=w973, "Data"=w970, "Address"=w971, "Logger"=w975) -> ("error out"=w972:errorcluster)  [unwired: 6 in, 1 out]
        n464 = call <vilib>:"Add State(s) to Queue__jki_lib_state_machine.vi"("State(s) in (\"\")"=w986) -> ("States Out"=w985:string)  [unwired: 14 in]
      }
    }
  }
  "Error Out" <- w2
  n465 = Unbundle By Name(w6) -> ("C.E."=→"Control Experiment":refnum<class "Control Experiment SM.lvclass">)
